vi "3_AdvancedDemo_MHT3.vi"() -> ()   [LabVIEW 2010]
uses:
  Types/MH_UIThread_Cmds.ctl
  _lib/PQ/MultiHarp/MH_InitInfo.ctl
  Types/MH_UIThread_Data.ctl
  Types/MH_InputChannel.ctl
  _lib/PQ/MultiHarp/MH_RefSource.ctl
  _lib/PQ/MultiHarp/mhlib_x86_x64_UIThread.llb/MH_DllPath_global.vi
  <vilib>/Utility/error.llb/DialogType.ctl
  Types/MH_DataProcThread_QCmds.ctl
  Types/MH_DataProcThread_QData.ctl
  Types/MH_VisThread_QCmds.ctl
  Types/MH_VisThread_QData.ctl
  Types/MH_VisThread_Data.ctl
  _lib/PQ/MultiHarp/MH_LibVersion_global.vi
  _lib/PQ/MultiHarp/MH_MeasMode.ctl
  Types/MH_SetInpChanData.ctl
  Types/MH_SetInpChanCmds.ctl
panel:
  in  "Settings":bool=TRUE
  in  "Run continuously":bool caption="Conti."
  in  "Start":bool
  in  "Scale":bool
  out "CountRates":i32[](graph)
  in  "AllChannels":T1={"Enable"=TRUE, "Offset"=0, "Level"=-100, "Edge"=0, "DeadTime"=1000, "UseDeadTime"=FALSE, "SetEnableAllChan"=TRUE, "SetEdgeAllChan"=TRUE, "SetLevelAllChan"=TRUE, "SetOffsetAllChan"=TRUE, "SetUseDTAllChan"=TRUE, "SetDeadTAllChan"=TRUE} {"DeadTime" min=800 max=160000 step=1; "Edge" items=["falling", "rising"]; "Offset" min=-100000 max=100000 step=5; "Level" min=-1200 max=1200 step=1}
  in  "HistoAcqTime":dbl=1.0 caption="Hist.Int.Time  s" min=0.1 max=360000.0 step=0.1
  in  "AcqTime":i32=360000000 caption="T3Acqu.       ms" min=1 max=360000 step=1
  in  "Binning":i32(ring) caption="Resol.            ps" items=["5", "10", "20", "40", "80", "160", "320", "640", "1280", "2560", "5120", "10240", "20480", "40960", "81920", "163840", "327680", "655360", "1310720", "2621440", "5242880", "10485760", "20971520", "41943040"]
  in  "HistoOffset":i32 caption="Offset            ns" min=0 max=100000000 step=1
  out "DeltaT":dbl=2.0479769602591973 caption="T.Tr.Resol.   ms" format="%.2f"
  in  "BitShift":i32=15 min=0 max=32 step=1
  in  "OvlLevel":u32=4294967295 caption="Ovl.Level" min=1024 max=65536 step=1024
  in  "StopOvl.":bool=TRUE
  out "TTraceGraph":T2(graph)={49.38852226226715, "Resolution"=0.00655367864414373, "Histogram"=[]}
  out "HistoGraph":cluster{dbl, "Resol":dbl, "Histos":u32[][]}(graph)={0.0, "Resol"=0.08, "Histos"=[]}
  in  "SyncDeadTime":i32=1000 caption="Dead T.   ps" min=800 max=160000 step=1
  in  "UseDeadTime":bool caption="Use DT."
  in  "SyncEdge":i32(ring) caption="Edge" items=["falling", "rising"]
  in  "SyncDivider":i32(ring) caption="Divider" items=["1", "2", "4", "8", "16"]
  in  "SyncOffset":i32 caption="Offset      ps" min=-100000 max=100000 step=5
  in  "SyncLevel":i32=-100 caption="Level      mV" min=-1200 max=1200 step=1
  in  "Channels":T3[](array[typedef])=[{"Name"="Inp.Chan 1", "Enable"=TRUE, "Edge"=0, "Level"=-100, "Offset"=0, "UseDeadTime"=FALSE, "DeadTime"=1000}, {"Name"="Inp.Chan 2", "Enable"=TRUE, "Edge"=0, "Level"=-100, "Offset"=0, "UseDeadTime"=FALSE, "DeadTime"=1000}, {"Name"="Inp.Chan 3", "Enable"=TRUE, "Edge"=0, "Level"=-100, "Offset"=0, "UseDeadTime"=FALSE, "DeadTime"=1000}, {"Name"="Inp.Chan 4", "Enable"=TRUE, "Edge"=0, "Level"=-100, "Offset"=0, "UseDeadTime"=FALSE, "DeadTime"=1000}, {"Name"="Inp.Chan 5", "Enable"=TRUE, "Edge"=0, "Level"=-100, "Offset"=0, "UseDeadTime"=FALSE, "DeadTime"=1000}, {"Name"="Inp.Chan 6", "Enable"=TRUE, "Edge"=0, "Level"=-100, "Offset"=0, "UseDeadTime"=FALSE, "DeadTime"=1000}, {"Name"="Inp.Chan 7", "Enable"=TRUE, "Edge"=0, "Level"=-100, "Offset"=0, "UseDeadTime"=FALSE, "DeadTime"=1000}, {"Name"="Inp.Chan 8", "Enable"=TRUE, "Edge"=0, "Level"=-100, "Offset"=0, "UseDeadTime"=FALSE, "DeadTime"=1000}, {"Name"="Inp.Chan 9", "Enable"=TRUE, "Edge"=0, "Level"=-100, "Offset"=0, "UseDeadTime"=FALSE, "DeadTime"=1000}, {"Name"="Inp.Chan 10", "Enable"=TRUE, "Edge"=0, "Level"=-100, "Offset"=0, "UseDeadTime"=FALSE, "DeadTime"=1000}, {"Name"="Inp.Chan 11", "Enable"=TRUE, "Edge"=0, "Level"=-100, "Offset"=0, "UseDeadTime"=FALSE, "DeadTime"=1000}, {"Name"="Inp.Chan 12", "Enable"=TRUE, "Edge"=0, "Level"=-100, "Offset"=0, "UseDeadTime"=FALSE, "DeadTime"=1000}, {"Name"="Inp.Chan 13", "Enable"=TRUE, "Edge"=0, "Level"=-100, "Offset"=0, "UseDeadTime"=FALSE, "DeadTime"=1000}, {"Name"="Inp.Chan 14", "Enable"=TRUE, "Edge"=0, "Level"=-100, "Offset"=0, "UseDeadTime"=FALSE, "DeadTime"=1000}, {"Name"="Inp.Chan 15", "Enable"=TRUE, "Edge"=0, "Level"=-100, "Offset"=0, "UseDeadTime"=FALSE, "DeadTime"=1000}, {"Name"="Inp.Chan 16", "Enable"=TRUE, "Edge"=0, "Level"=-100, "Offset"=0, "UseDeadTime"=FALSE, "DeadTime"=1000}, {"Name"="Inp.Chan 17", "Enable"=TRUE, "Edge"=0, "Level"=-100, "Offset"=0, "UseDeadTime"=FALSE, "DeadTime"=1000}, {"Name"="Inp.Chan 18", "Enable"=TRUE, "Edge"=0, "Level"=-100, "Offset"=0, "UseDeadTime"=FALSE, "DeadTime"=1000}, {"Name"="Inp.Chan 19", "Enable"=TRUE, "Edge"=0, "Level"=-100, "Offset"=0, "UseDeadTime"=FALSE, "DeadTime"=1000}, {"Name"="Inp.Chan 20", "Enable"=TRUE, "Edge"=0, "Level"=-100, "Offset"=0, "UseDeadTime"=FALSE, "DeadTime"=1000}, {"Name"="Inp.Chan 21", "Enable"=TRUE, "Edge"=0, "Level"=-100, "Offset"=0, "UseDeadTime"=FALSE, "DeadTime"=1000}, {"Name"="Inp.Chan 22", "Enable"=TRUE, "Edge"=0, "Level"=-100, "Offset"=0, "UseDeadTime"=FALSE, "DeadTime"=1000}, {"Name"="Inp.Chan 23", "Enable"=TRUE, "Edge"=0, "Level"=-100, "Offset"=0, "UseDeadTime"=FALSE, "DeadTime"=1000}, {"Name"="Inp.Chan 24", "Enable"=TRUE, "Edge"=0, "Level"=-100, "Offset"=0, "UseDeadTime"=FALSE, "DeadTime"=1000}, {"Name"="Inp.Chan 25", "Enable"=TRUE, "Edge"=0, "Level"=-100, "Offset"=0, "UseDeadTime"=FALSE, "DeadTime"=1000}, {"Name"="Inp.Chan 26", "Enable"=TRUE, "Edge"=0, "Level"=-100, "Offset"=0, "UseDeadTime"=FALSE, "DeadTime"=1000}, {"Name"="Inp.Chan 27", "Enable"=TRUE, "Edge"=0, "Level"=-100, "Offset"=0, "UseDeadTime"=FALSE, "DeadTime"=1000}, {"Name"="Inp.Chan 28", "Enable"=TRUE, "Edge"=0, "Level"=-100, "Offset"=0, "UseDeadTime"=FALSE, "DeadTime"=1000}, {"Name"="Inp.Chan 29", "Enable"=TRUE, "Edge"=0, "Level"=-100, "Offset"=0, "UseDeadTime"=FALSE, "DeadTime"=1000}, {"Name"="Inp.Chan 30", "Enable"=TRUE, "Edge"=0, "Level"=-100, "Offset"=0, "UseDeadTime"=FALSE, "DeadTime"=1000}, {"Name"="Inp.Chan 31", "Enable"=TRUE, "Edge"=0, "Level"=-100, "Offset"=0, "UseDeadTime"=FALSE, "DeadTime"=1000}, {"Name"="Inp.Chan 32", "Enable"=TRUE, "Edge"=0, "Level"=-100, "Offset"=0, "UseDeadTime"=FALSE, "DeadTime"=1000}, {"Name"="Inp.Chan 33", "Enable"=TRUE, "Edge"=0, "Level"=-100, "Offset"=0, "UseDeadTime"=FALSE, "DeadTime"=1000}, {"Name"="Inp.Chan 34", "Enable"=TRUE, "Edge"=0, "Level"=-100, "Offset"=0, "UseDeadTime"=FALSE, "DeadTime"=1000}, {"Name"="Inp.Chan 35", "Enable"=TRUE, "Edge"=0, "Level"=-100, "Offset"=0, "UseDeadTime"=FALSE, "DeadTime"=1000}, {"Name"="Inp.Chan 36", "Enable"=TRUE, "Edge"=0, "Level"=-100, "Offset"=0, "UseDeadTime"=FALSE, "DeadTime"=1000}, {"Name"="Inp.Chan 37", "Enable"=TRUE, "Edge"=0, "Level"=-100, "Offset"=0, "UseDeadTime"=FALSE, "DeadTime"=1000}, {"Name"="Inp.Chan 38", "Enable"=TRUE, "Edge"=0, "Level"=-100, "Offset"=0, "UseDeadTime"=FALSE, "DeadTime"=1000}, {"Name"="Inp.Chan 39", "Enable"=TRUE, "Edge"=0, "Level"=-100, "Offset"=0, "UseDeadTime"=FALSE, "DeadTime"=1000}, {"Name"="Inp.Chan 40", "Enable"=TRUE, "Edge"=0, "Level"=-100, "Offset"=0, "UseDeadTime"=FALSE, "DeadTime"=1000}, {"Name"="Inp.Chan 41", "Enable"=TRUE, "Edge"=0, "Level"=-100, "Offset"=0, "UseDeadTime"=FALSE, "DeadTime"=1000}, {"Name"="Inp.Chan 42", "Enable"=TRUE, "Edge"=0, "Level"=-100, "Offset"=0, "UseDeadTime"=FALSE, "DeadTime"=1000}, {"Name"="Inp.Chan 43", "Enable"=TRUE, "Edge"=0, "Level"=-100, "Offset"=0, "UseDeadTime"=FALSE, "DeadTime"=1000}, {"Name"="Inp.Chan 44", "Enable"=TRUE, "Edge"=0, "Level"=-100, "Offset"=0, "UseDeadTime"=FALSE, "DeadTime"=1000}, {"Name"="Inp.Chan 45", "Enable"=TRUE, "Edge"=0, "Level"=-100, "Offset"=0, "UseDeadTime"=FALSE, "DeadTime"=1000}, {"Name"="Inp.Chan 46", "Enable"=TRUE, "Edge"=0, "Level"=-100, "Offset"=0, "UseDeadTime"=FALSE, "DeadTime"=1000}, {"Name"="Inp.Chan 47", "Enable"=TRUE, "Edge"=0, "Level"=-100, "Offset"=0, "UseDeadTime"=FALSE, "DeadTime"=1000}, {"Name"="Inp.Chan 48", "Enable"=TRUE, "Edge"=0, "Level"=-100, "Offset"=0, "UseDeadTime"=FALSE, "DeadTime"=1000}, {"Name"="Inp.Chan 49", "Enable"=TRUE, "Edge"=0, "Level"=-100, "Offset"=0, "UseDeadTime"=FALSE, "DeadTime"=1000}, {"Name"="Inp.Chan 50", "Enable"=TRUE, "Edge"=0, "Level"=-100, "Offset"=0, "UseDeadTime"=FALSE, "DeadTime"=1000}, {"Name"="Inp.Chan 51", "Enable"=TRUE, "Edge"=0, "Level"=-100, "Offset"=0, "UseDeadTime"=FALSE, "DeadTime"=1000}, {"Name"="Inp.Chan 52", "Enable"=TRUE, "Edge"=0, "Level"=-100, "Offset"=0, "UseDeadTime"=FALSE, "DeadTime"=1000}, {"Name"="Inp.Chan 53", "Enable"=TRUE, "Edge"=0, "Level"=-100, "Offset"=0, "UseDeadTime"=FALSE, "DeadTime"=1000}, {"Name"="Inp.Chan 54", "Enable"=TRUE, "Edge"=0, "Level"=-100, "Offset"=0, "UseDeadTime"=FALSE, "DeadTime"=1000}, {"Name"="Inp.Chan 55", "Enable"=TRUE, "Edge"=0, "Level"=-100, "Offset"=0, "UseDeadTime"=FALSE, "DeadTime"=1000}, {"Name"="Inp.Chan 56", "Enable"=TRUE, "Edge"=0, "Level"=-100, "Offset"=0, "UseDeadTime"=FALSE, "DeadTime"=1000}, {"Name"="Inp.Chan 57", "Enable"=TRUE, "Edge"=0, "Level"=-100, "Offset"=0, "UseDeadTime"=FALSE, "DeadTime"=1000}, {"Name"="Inp.Chan 58", "Enable"=TRUE, "Edge"=0, "Level"=-100, "Offset"=0, "UseDeadTime"=FALSE, "DeadTime"=1000}, {"Name"="Inp.Chan 59", "Enable"=TRUE, "Edge"=0, "Level"=-100, "Offset"=0, "UseDeadTime"=FALSE, "DeadTime"=1000}, {"Name"="Inp.Chan 60", "Enable"=TRUE, "Edge"=0, "Level"=-100, "Offset"=0, "UseDeadTime"=FALSE, "DeadTime"=1000}, {"Name"="Inp.Chan 61", "Enable"=TRUE, "Edge"=0, "Level"=-100, "Offset"=0, "UseDeadTime"=FALSE, "DeadTime"=1000}, {"Name"="Inp.Chan 62", "Enable"=TRUE, "Edge"=0, "Level"=-100, "Offset"=0, "UseDeadTime"=FALSE, "DeadTime"=1000}, {"Name"="Inp.Chan 63", "Enable"=TRUE, "Edge"=0, "Level"=-100, "Offset"=0, "UseDeadTime"=FALSE, "DeadTime"=1000}, {"Name"="Inp.Chan 64", "Enable"=TRUE, "Edge"=0, "Level"=-100, "Offset"=0, "UseDeadTime"=FALSE, "DeadTime"=1000}] {"DeadTime" min=800 max=160000 step=1; "Edge" items=["falling", "rising"]; "Offset" min=-100000 max=100000 step=5; "Level" min=-1200 max=1200 step=1}
  out "SyncRate":string="Sync Rate: 16000190 cps\n"
  out "OverRun":bool caption="Overrun:"
  out "Status":string="Elements in Q: 0"
  # "All Channels"
  # "Acquisition"
  # "Sync"
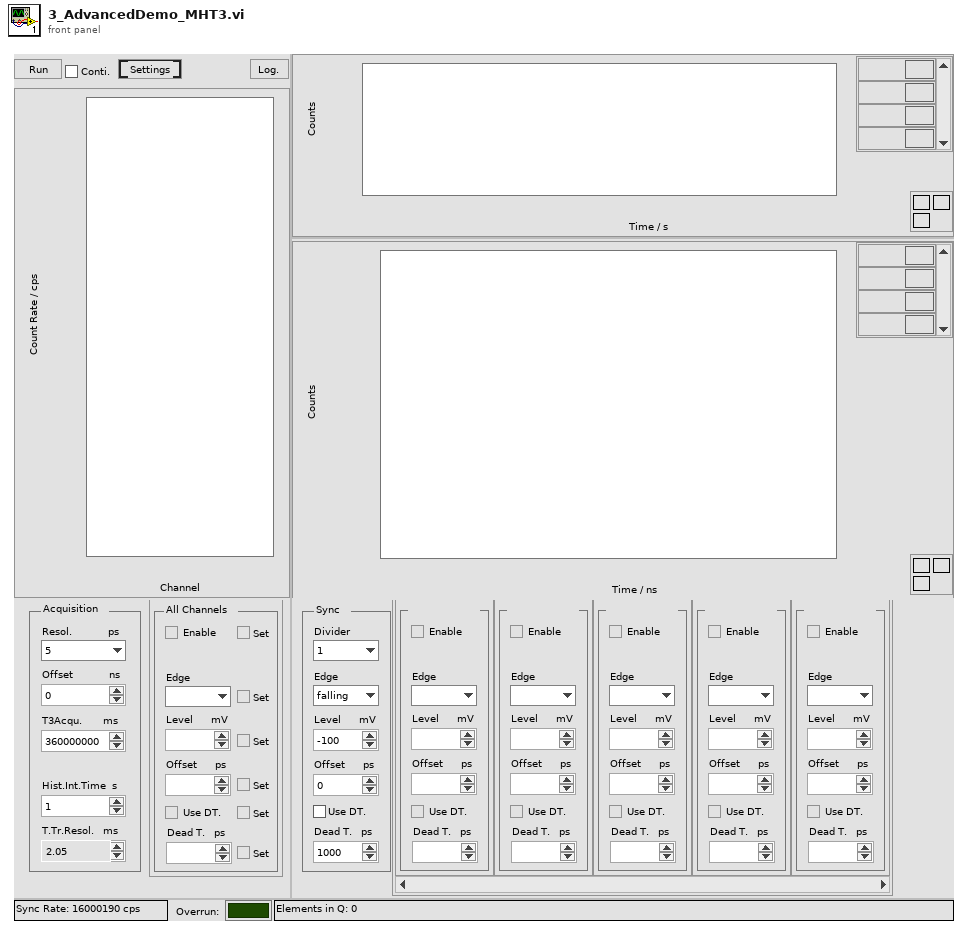
[diagram p1: front panel]
types:
  T1 = cluster{"Enable":bool, "Offset":i32, "Level":i32, "Edge":i32, "DeadTime":i32, "UseDeadTime":bool, "SetEnableAllChan":bool, "SetEdgeAllChan":bool, "SetLevelAllChan":bool, "SetOffsetAllChan":bool, "SetUseDTAllChan":bool, "SetDeadTAllChan":bool}
  T2 = cluster{dbl, "Resolution":dbl, "Histogram":u32[][]}
  T3 = typedef "MH_InputChannel.ctl" = cluster{"Name":string, "Enable":bool, "Edge":i32, "Level":i32, "Offset":i32, "UseDeadTime":bool, "DeadTime":i32}
  T4 = typedef "MH_DataProcThread_QCmds.ctl" = enum16{"Exit", "Proc", "Init", "SetShift", "SetNumChannels", "SetHistAcqTime"}
  T5 = typedef "MH_VisThread_Data.ctl" = cluster{"Resol":dbl, "DeltaT":dbl, "NumChannels":i32}
  T6 = typedef "MH_VisThread_QData.ctl" = cluster{"Histos":u32[][], "Cmd":T7, "TimeTrace":u32[][], "Bin":i32, "Total bin":u64, "Status":string, "Resol":dbl, "DeltaT":dbl, "nChannels":i32}
  T7 = typedef "MH_VisThread_QCmds.ctl" = enum16{"_none_", "Resol", "nChannels", "DeltaT", "Histo", "TTrace", "Status"}
  T8 = typedef "MH_DataProcThread_QData.ctl" = cluster{"Cmd":T4, "nActual":i32, "Buffer":u32[], "TickCount":u32, "Param":i32}
  T9 = typedef "MH_UIThread_Data.ctl" = cluster{"Init Info":T10, "DevIdx":i32, "SyncDivider":i32, "SyncOffset":i32, "SyncLevel":i32, "Channels":T3[], "CurrentChannels":i32[], "AcqTime":i32, "Binning":i32, "HistoOffset":i32, "HistoLen":i32, "StopOvl.":bool, "OvlLevel":u32, "SyncEdge":i32, "StartMeas":bool, "HistoLength":i32, "Resolution":dbl, "Run cont.":bool, "Status":string, "SyncRate":i32, "BitShift":i32, "HistoAcqTime":dbl, "SyncRateStart":i32, "UseDeadTime":bool, "SyncDeadTime":i32, "SetInpChan":T11[]}
  T10 = typedef "MH_InitInfo.ctl" = cluster{"Library Version":string, "Serial No.":string, "Model":string, "Partnum":string, "Version":string, "features":i32, "nchannels":i32, "Base Resolution":dbl, "Bin Steps":i32}
  T11 = typedef "MH_SetInpChanData.ctl" = cluster{"Channel":i32, "Cmds":T12[], "Changed":cluster{"Name":bool, "Enable":bool, "Edge":bool, "Level":bool, "Offset":bool, "UseDeadTime":bool, "DeadTime":bool}}
  T12 = typedef "MH_SetInpChanCmds.ctl" = enum16{"SetInpChanEnable", "SetInpChanOffset", "SetInpChanDeadTime", "SetInpChanTrg"}
  T13 = typedef "MH_UIThread_Cmds.ctl" = enum16{"Idle", "Init", "SetInpChan", "SetSyncDivider", "SetSyncTrg", "SetSyncOffset", "SetSyncDeadTime", "SetBinning", "SetHistoOffset", "SetHistoLen", "SetStopOvl", "SetBitShift", "SetHistoAcqTime", "GetRates", "GetAllRates", "StartMeas", "StopMeas", "AbortMeas", "GetResolution", "GetHistos", "GetAllHistos", "ReadFiFo", "WriteStatus", "Resize", "EnableControls", "DisableControls", "Error", "Exit"}
  T14 = enum8{"Enabled", "Disabled", "Disabled and Grayed Out"}
  T15 = cluster{"[0]":bool, "[1]":bool, "[2]":bool, "[3]":bool, "[4]":bool, "[5]":bool}
  T16 = typedef "MH_MeasMode.ctl" = i32
  T17 = typedef "MH_RefSource.ctl" = enum16{"INTERNAL", "EXTERNAL_10MHZ", "WR_MASTER_GENERIC", "WR_SLAVE_GENERIC", "WR_GRANDM_GENERIC", "EXTN_GPS_PPS", "EXTN_GPS_PPS_UART", "WR_MASTER_MHARP", "WR_SLAVE_MHARP", "WR_GRANDM_MHARP"}
  T18 = typedef "DialogType.ctl" = u16
  T19 = cluster{"T0":dbl, "dt":dbl, "TimeTrace_out":u32[][]}
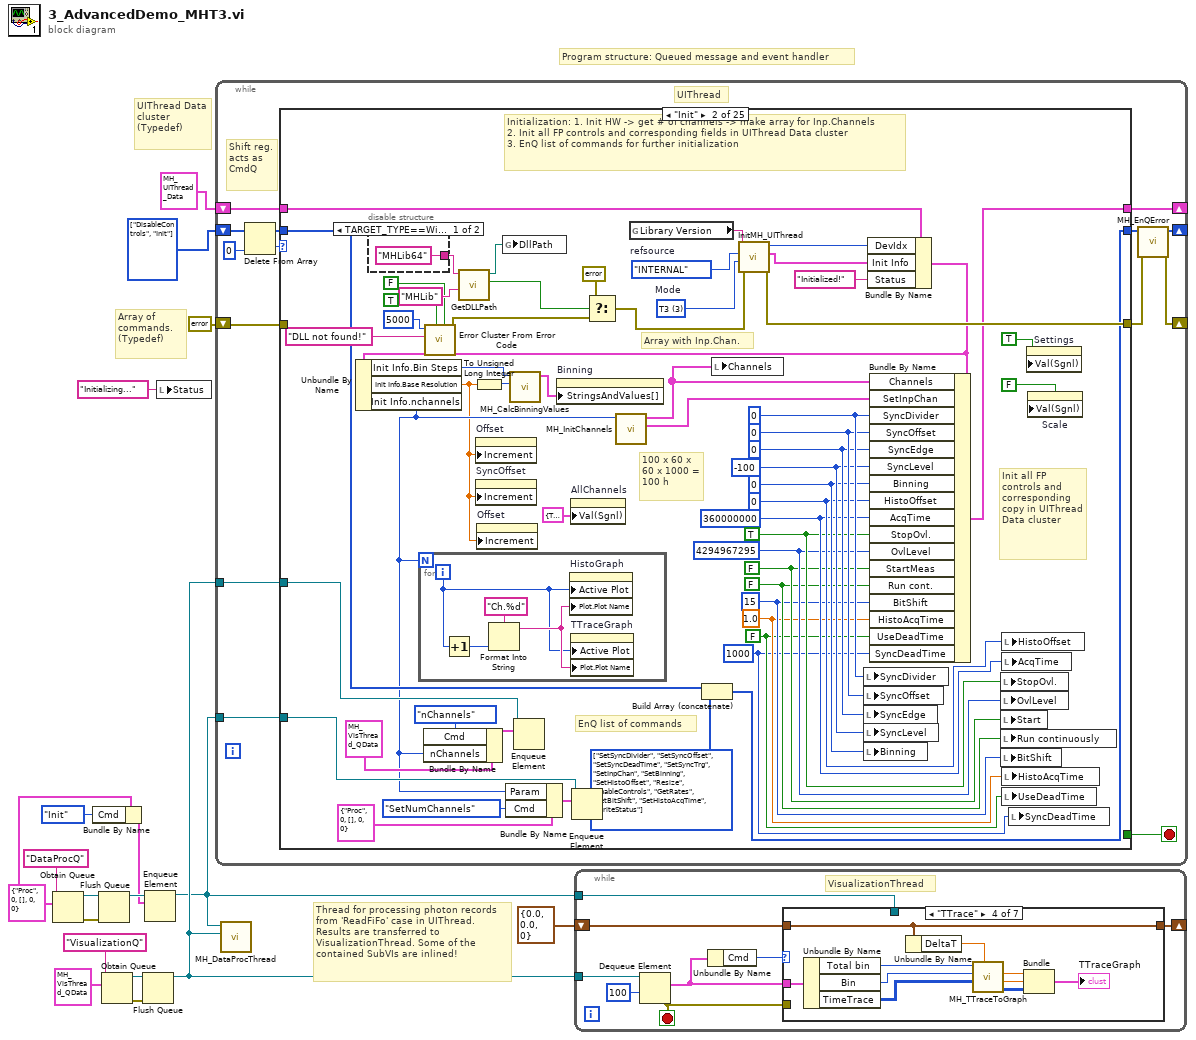
[diagram p0: block diagram]
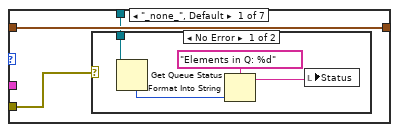
[diagram p2: hidden frame]
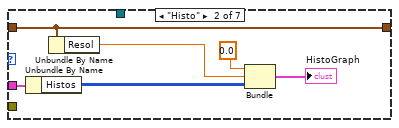
[diagram p4: hidden frame]
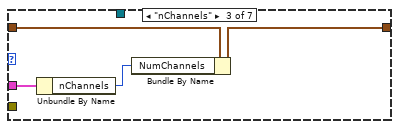
[diagram p5: hidden frame]
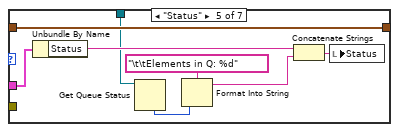
[diagram p6: hidden frame]
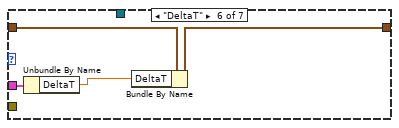
[diagram p7: hidden frame]
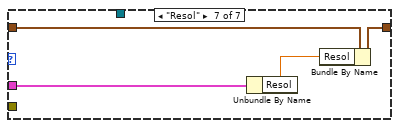
[diagram p8: hidden frame]
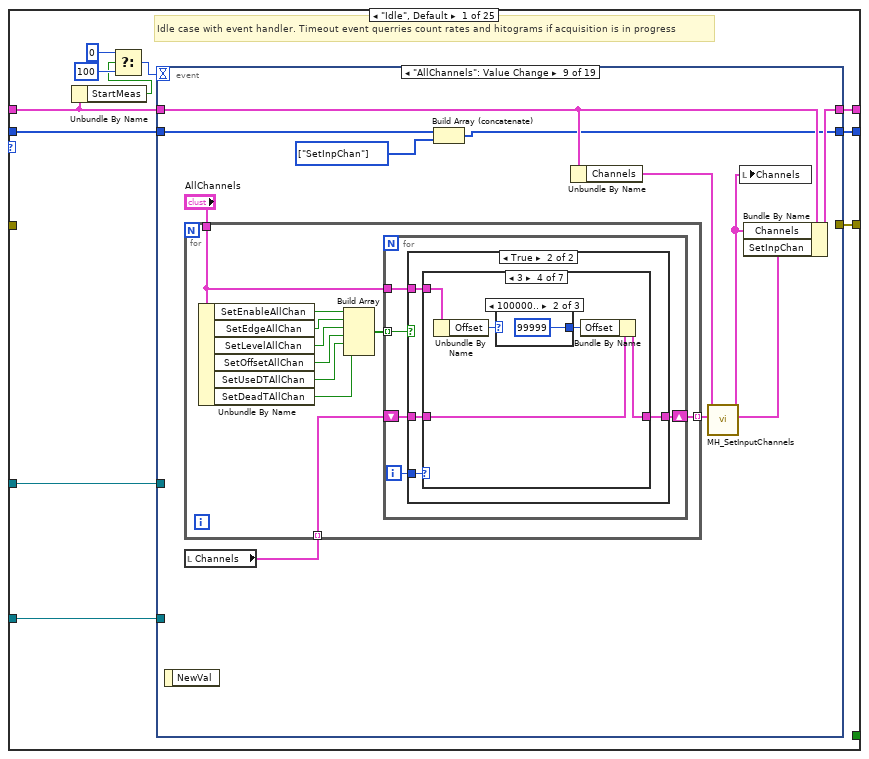
[diagram p9: hidden frame]
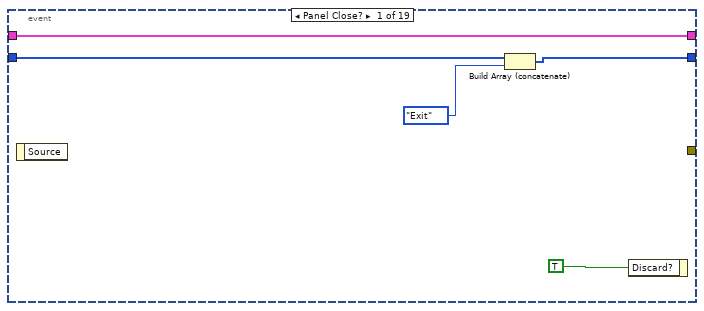
[diagram p10: hidden frame]
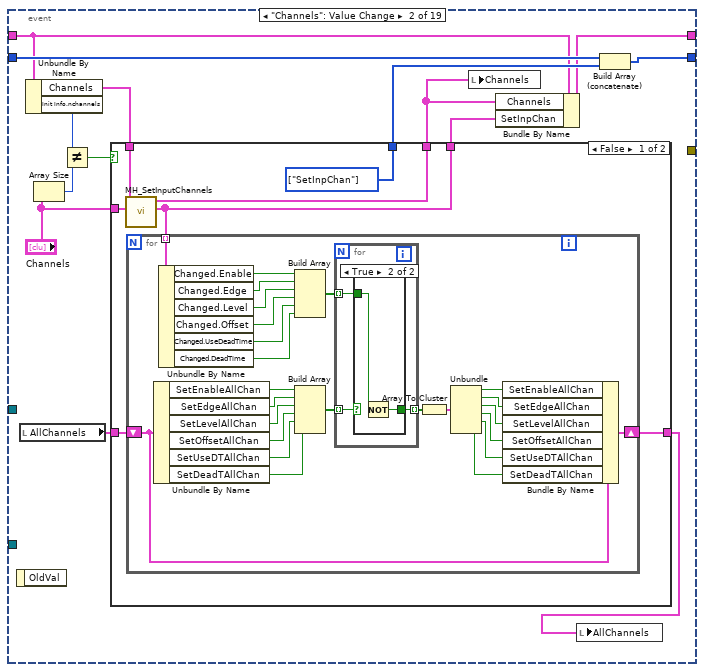
[diagram p11: hidden frame]
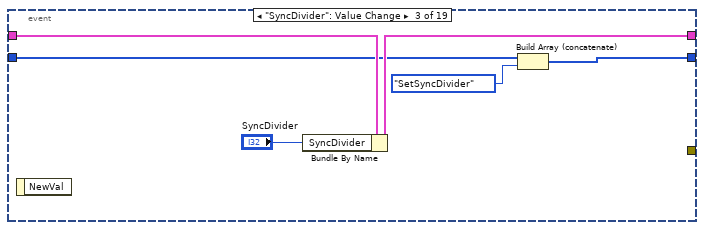
[diagram p14: hidden frame]
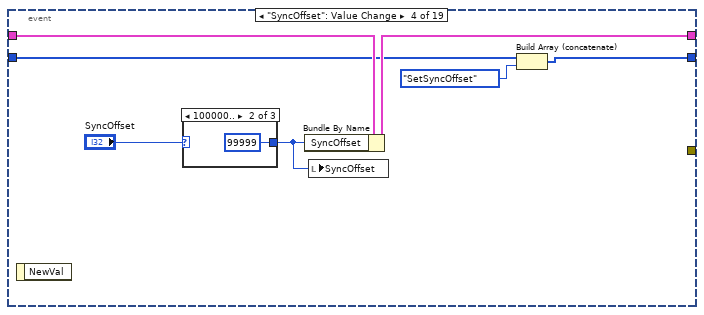
[diagram p15: hidden frame]
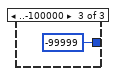
[diagram p17: hidden frame]
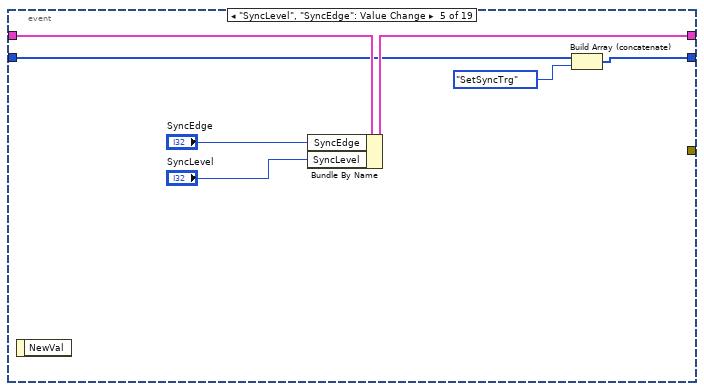
[diagram p18: hidden frame]
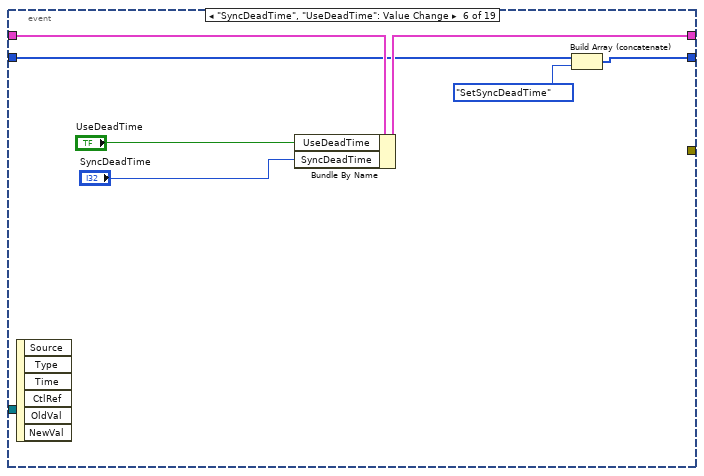
[diagram p19: hidden frame]
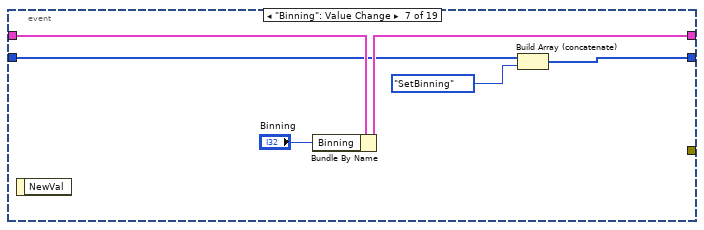
[diagram p20: hidden frame]
diagram:
  w4 = T8 {"Cmd"=enum."Proc", "nActual"=0, "Buffer"=[], "TickCount"=0, "Param"=0} ("MH_DataProcThread_QData")
  w17 = T13[] [enum."DisableControls", enum."Init"] items=["Idle", "Init", "SetInpChan", "SetSyncDivider", "SetSyncTrg", "SetSyncOffset", "SetSyncDeadTime", "SetBinning", "SetHistoOffset", "SetHistoLen", "SetStopOvl", "SetBitShift", "SetHistoAcqTime", "GetRates", "GetAllRates", "StartMeas", "StopMeas", "AbortMeas", "GetResolution", "GetHistos", "GetAllHistos", "ReadFiFo", "WriteStatus", "Resize", "EnableControls", "DisableControls", "Error", "Exit"]
  # "Thread for processing photon records from 'ReadFiFo' case in UIThread. Results are transferred to VisualizationThread. Some of the contained SubVIs are inlined!"
  # "Array of commands.\n(Typedef)"
  # "Program structure: Queued message and event handler"
  # "UIThread Data cluster\n(Typedef)"
  n1 = Obtain Queue(name (unnamed)="DataProcQ", element data type=w4) -> (queue out=w14:refnum<queue>, error out=w13:errorcluster)  [unwired: 3 in, 1 out]
  n2 = Bundle By Name(cluster=w4, "Cmd"=MH_DataProcThread_QCmds."Init") -> (w2:T8)
  n3 = Flush Queue(queue=w14, error in (no error)=w13) -> (queue out=w5:refnum<queue>)  [unwired: 2 out]
  n4 = Obtain Queue(name (unnamed)="VisualizationQ", element data type=T6 {"Histos"=[], "Cmd"=enum."_none_", "TimeTrace"=[], "Bin"=0, "Total bin"=0, "Status"="", "Resol"=0.0, "DeltaT"=0.0, "nChannels"=0} ("MH_GUIThread_QData")) -> (queue out=w12:refnum<queue>, error out=w11:errorcluster)  [unwired: 3 in, 1 out]
  n5 = Flush Queue(queue=w12, error in (no error)=w11) -> (queue out=w7:refnum<queue>)  [unwired: 2 out]
  n6 = Enqueue Element(queue=w5, element=w2) -> (queue out=w1:refnum<queue>)  [unwired: 2 in, 2 out]
  n7 = local write "Status"("Initializing..." ("Status")) -> ()
  n8 = while {
    shift-right: [w21] -> _
    shift-left: w17 -> [w28]
    shift-right: [w31] -> _
    shift-left: T9 {"Init Info"={"Library Version"="", "Serial No."="", "Model"="", "Partnum"="", "Version"="", "features"=0, "nchannels"=0, "Base Resolution"=0.0, "Bin Steps"=0}, "DevIdx"=0, "SyncDivider"=1, "SyncOffset"=0, "SyncLevel"=50, "Channels"=[], "CurrentChannels"=[], "AcqTime"=1, "Binning"=1, "HistoOffset"=1, "HistoLen"=1024, "StopOvl."=FALSE, "OvlLevel"=1024, "SyncEdge"=10, "StartMeas"=FALSE, "HistoLength"=0, "Resolution"=0.0, "Run cont."=FALSE, "Status"="", "SyncRate"=0, "BitShift"=0, "HistoAcqTime"=0.0, "SyncRateStart"=0, "UseDeadTime"=FALSE, "SyncDeadTime"=800, "SetInpChan"=[]} -> [w30]
    shift-right: [w23] -> _
    shift-left: errorcluster {"status"=FALSE, "code"=0, "source"=""} ("error IO") -> [w29]
    tunnel: w1 -> [w20]
    tunnel: w7 -> [w19]
    stop <- w32 stop-if-true
    # "Shift reg.\nacts as\nCmdQ"
    # "UIThread"
    n9 = Delete From Array(array=w28, index=0) -> (deleted portion=w26:T13, array with subset deleted=w25:T13[])  [unwired: 1 in]
    n10 = case shown="\"Init\"" w26 {
      tunnel: [w43 w359 w377 w439 w448 w460 w466 w473 w481 w488 w508 w520 w523 w595 w618 w623 w636 w653 w654 w680 w693 w700 w712 w718 w724] -> w22
      tunnel: [_ _ _ _ _ _ _ _ _ _ _ _ _ _ _ _ _ _ _ _ _ _ _ _ TRUE] -> w32
      tunnel: [w42 w340 w378 w441 w449 w461 w470 w477 w482 w489 w493 w510 w532 w587 w610 w626 w638 w649 w664 w679 w681 w699 w711 w719 w727] -> w31
      tunnel: w30 -> [w39 w345 w378 w441 w449 w461 w470 w477 w482 w489 w493 w510 w522 w588 w611 w627 w639 w650 w664 w679 w681 w699 w711 w719 w727]
      tunnel: [w40 w362 w372 w437 w447 w459 w469 w476 w480 w487 _ _ w528 w594 w621 w629 w641 w651 w659 _ _ _ _ _ w725] -> w24
      tunnel: w29 -> [_ _ _ _ _ _ _ _ _ _ _ _ _ _ _ _ _ _ _ _ _ _ _ w720 _]
      tunnel: w25 -> [w41 w361 w377 w439 w448 w460 w466 w472 w481 w488 w508 w520 w524 w595 w619 w624 w636 w653 w655 w680 w693 w700 w712 _ w724]
      tunnel: w20 -> [w34 w338 _ _ _ _ _ _ _ _ w494 w511 _ _ w615 _ _ _ w656 _ _ _ _ _ w723]
      tunnel: w19 -> [w33 w331 _ _ _ _ _ _ _ _ w495 _ _ _ _ _ _ w646 _ _ _ _ _ _ w722]
      frame "Idle", Default {
        # "Idle case with event handler. Timeout event querries count rates and hitograms if acquisition is in progress"
        n11 = Unbundle By Name(w39) -> ("StartMeas"=w37:bool)
        n12 = Select(t=0, s=w37, f=100) -> (s? t:f=w36:i32)
        n13 = event shown="[8] \"AllChannels\": Value Change" {
          selector: _ -> [_ _ _ _ _ _ _ _ _ _ _ _ _ _ _ _ _ _ _]
          dyn-events: _ -> [_ _ _ _ _ _ _ _ _ _ _ _ _ _ _ _ _ _ _]
          timeout: w36 -> [_ _ _ _ _ _ _ _ _ _ _ _ _ _ _ _ _ _ _]
          tunnel: [w44 w61 w103 w111 w120 w128 w134 w140 w145 w205 w210 w217 w232 w250 w262 w280 w286 w294 w304] -> w43
          tunnel: [w47 w53 w107 w114 w124 w131 w137 w143 w150 w207 w213 w220 w231 w254 w261 w278 w285 w293 w307] -> w42
          tunnel: w39 -> [w47 w54 w108 w115 w125 w132 w138 w144 w151 w208 w214 w221 w231 w255 w259 w279 w285 w293 w307]
          tunnel: w41 -> [w46 w62 w105 w113 w122 w130 w136 w142 w146 w205 w211 w219 w233 w251 w263 w280 w286 w294 w305]
          tunnel: [_ _ _ _ _ _ _ _ _ _ _ _ w227 _ _ _ _ _ _] -> w40
          tunnel: w34 -> [_ _ _ _ _ _ _ _ _ _ _ _ _ _ _ _ _ _ _]
          tunnel: w33 -> [_ _ _ _ _ _ _ _ _ _ _ _ _ _ _ _ _ _ _]
          event Panel Close? {
            n14 = event-data() -> ()  [unwired: 1 in, 1 out]
            n15 = Build Array (concatenate)(w46, MH_UIThread_Cmds."Exit") -> (w44:T13[])
            n16 = event-data("Discard?"=TRUE) -> ()  [unwired: 1 in, 1 out]
          }
          event "Channels": Value Change {
            n17 = event-data() -> ()  [unwired: 1 in, 1 out]
            n18 = local read "AllChannels"() -> (w49:T1)
            n19 = Unbundle By Name(w54) -> ("Channels"=w56:T3[], "Init Info.nchannels"=w58:i32)
            n20 = Array Size(array="Channels") -> (size(s)=w59:i32)
            n21 = Not Equal?(x=w58, y=w59) -> (x != y?=w57:bool)
            n22 = case shown="False" w57 {
              tunnel: "Channels" -> [w68 _]
              tunnel: [w67 w102] -> w51
              tunnel: w56 -> [w69 w102]
              tunnel: [w65 _] -> w52
              tunnel: [w66 _] -> w55
              tunnel: w49 -> [w64 w101]
              tunnel: [w63 w101] -> w50
              frame False {
                w66 = T13[] [enum."SetInpChan"] items=["Idle", "Init", "SetInpChan", "SetSyncDivider", "SetSyncTrg", "SetSyncOffset", "SetSyncDeadTime", "SetBinning", "SetHistoOffset", "SetHistoLen", "SetStopOvl", "SetBitShift", "SetHistoAcqTime", "GetRates", "GetAllRates", "StartMeas", "StopMeas", "AbortMeas", "GetResolution", "GetHistos", "GetAllHistos", "ReadFiFo", "WriteStatus", "Resize", "EnableControls", "DisableControls", "Error", "Exit"] ("array")
                n23 = call "MH_SetInputChannels.vi"("Channels new"=w68, "Channels old"=w69) -> ("SetInpChan"=w65:T11[], "Channels"=w67:T3[])  [unwired: 8 in]
                n24 = for {
                  tunnel: w65 -> [w94] mode=indexing
                  shift-right: [w76] -> w63
                  shift-left: w64 -> [w78]
                  n25 = Unbundle By Name(w78) -> ("SetEnableAllChan"=w87:bool, "SetEdgeAllChan"=w86:bool, "SetLevelAllChan"=w85:bool, "SetOffsetAllChan"=w84:bool, "SetUseDTAllChan"=w83:bool, "SetDeadTAllChan"=w82:bool)
                  n26 = Unbundle By Name(w94) -> ("Changed.Enable"=w93:bool, "Changed.Edge"=w92:bool, "Changed.Level"=w91:bool, "Changed.Offset"=w90:bool, "Changed.UseDeadTime"=w89:bool, "Changed.DeadTime"=w88:bool)
                  n27 = Build Array(w93, w92, w91, w90, w89, w88) -> (w80:bool[])
                  n28 = Build Array(w87, w86, w85, w84, w83, w82) -> (w81:bool[])
                  n29 = for {
                    tunnel: w81 -> [w97] mode=indexing
                    tunnel: w80 -> [w95] mode=indexing
                    tunnel: [w96] -> w79 mode=indexing
                    n30 = case shown="True" w97 {
                      selector: w97 -> [w98 _]
                      tunnel: [w98 w99] -> w96
                      tunnel: w95 -> [_ w100]
                      frame False {
                      }
                      frame True {
                        n31 = Not(x=w100) -> (.not. x?=w99:bool)
                      }
                    }
                  }
                  n32 = Array To Cluster(array=w79) -> (cluster=w77:T15)
                  n33 = Unbundle(w77) -> ("[0]"=w75:bool, "[1]"=w74:bool, "[2]"=w73:bool, "[3]"=w72:bool, "[4]"=w71:bool, "[5]"=w70:bool)
                  n34 = Bundle By Name(cluster=w78, "SetEnableAllChan"=w75, "SetEdgeAllChan"=w74, "SetLevelAllChan"=w73, "SetOffsetAllChan"=w72, "SetUseDTAllChan"=w71, "SetDeadTAllChan"=w70) -> (w76:T1)
                }
              }
              frame True {
              }
            }
            n35 = local write "Channels"(w51) -> ()
            n36 = Bundle By Name(cluster=w54, "Channels"=w51, "SetInpChan"=w52) -> (w53:T9)
            n37 = local write "AllChannels"(w50) -> ()
            n38 = Build Array (concatenate)(w62, w55) -> (w61:T13[])
          }
          event "SyncDivider": Value Change {
            n39 = event-data() -> ()  [unwired: 1 in, 1 out]
            n40 = Bundle By Name(cluster=w108, "SyncDivider"="SyncDivider") -> (w107:T9)
            n41 = Build Array (concatenate)(w105, MH_UIThread_Cmds."SetSyncDivider") -> (w103:T13[])
          }
          event "SyncOffset": Value Change {
            n42 = event-data() -> ()  [unwired: 1 in, 1 out]
            n43 = case shown="100000.." "SyncOffset" {
              selector: "SyncOffset" -> [w116 _ _]
              tunnel: [w116 99999 ("SyncOffset") -99999 ("SyncOffset")] -> w109
              frame Default {
              }
              frame 100000.. {
              }
              frame ..-100000 {
              }
            }
            n44 = Bundle By Name(cluster=w115, "SyncOffset"=w109) -> (w114:T9)
            n45 = local write "SyncOffset"(w109) -> ()
            n46 = Build Array (concatenate)(w113, MH_UIThread_Cmds."SetSyncOffset") -> (w111:T13[])
          }
          event "SyncLevel", "SyncEdge": Value Change {
            n47 = event-data() -> ()  [unwired: 1 in, 1 out]
            n48 = Bundle By Name(cluster=w125, "SyncEdge"="SyncEdge", "SyncLevel"="SyncLevel") -> (w124:T9)
            n49 = Build Array (concatenate)(w122, MH_UIThread_Cmds."SetSyncTrg") -> (w120:T13[])
          }
          event "SyncDeadTime", "UseDeadTime": Value Change {
            n50 = event-data() -> ()  [unwired: 1 in, 6 out]
            n51 = Bundle By Name(cluster=w132, "UseDeadTime"="UseDeadTime", "SyncDeadTime"="SyncDeadTime") -> (w131:T9)
            n52 = Build Array (concatenate)(w130, MH_UIThread_Cmds."SetSyncDeadTime") -> (w128:T13[])
          }
          event "Binning": Value Change {
            n53 = event-data() -> ()  [unwired: 1 in, 1 out]
            n54 = Bundle By Name(cluster=w138, "Binning"="Binning") -> (w137:T9)
            n55 = Build Array (concatenate)(w136, MH_UIThread_Cmds."SetBinning") -> (w134:T13[])
          }
          event "HistoOffset": Value Change {
            n56 = event-data() -> ()  [unwired: 1 in, 1 out]
            n57 = Bundle By Name(cluster=w144, "HistoOffset"="HistoOffset") -> (w143:T9)
            n58 = Build Array (concatenate)(w142, MH_UIThread_Cmds."SetHistoOffset") -> (w140:T13[])
          }
          event "AllChannels": Value Change {
            w147 = T13[] [enum."SetInpChan"] items=["Idle", "Init", "SetInpChan", "SetSyncDivider", "SetSyncTrg", "SetSyncOffset", "SetSyncDeadTime", "SetBinning", "SetHistoOffset", "SetHistoLen", "SetStopOvl", "SetBitShift", "SetHistoAcqTime", "GetRates", "GetAllRates", "StartMeas", "StopMeas", "AbortMeas", "GetResolution", "GetHistos", "GetAllHistos", "ReadFiFo", "WriteStatus", "Resize", "EnableControls", "DisableControls", "Error", "Exit"] ("array")
            n59 = event-data() -> ()  [unwired: 1 in, 1 out]
            n60 = local read "Channels"() -> (w154:T3[])
            n61 = for {
              tunnel: w154 -> [w158] mode=indexing
              tunnel: "AllChannels" -> [w157]
              tunnel: [w156] -> w153 mode=indexing
              n62 = Unbundle By Name(w157) -> ("SetEnableAllChan"=w159:bool, "SetEdgeAllChan"=w160:bool, "SetLevelAllChan"=w161:bool, "SetOffsetAllChan"=w162:bool, "SetUseDTAllChan"=w163:bool, "SetDeadTAllChan"=w164:bool)
              n63 = Build Array(w159, w160, w161, w162, w163, w164) -> (w165:bool[])
              n64 = for {
                tunnel: w165 -> [w170] mode=indexing
                shift-right: [w167] -> w156
                shift-left: w158 -> [w168]
                tunnel: w157 -> [w166]
                i -> [w169]
                n65 = case shown="True" w170 {
                  tunnel: w169 -> [_ w175]
                  tunnel: w166 -> [_ w174]
                  tunnel: w168 -> [w171 w173]
                  tunnel: [w171 w172] -> w167
                  frame False {
                  }
                  frame True {
                    n66 = case shown="3" w175 {
                      tunnel: w174 -> [w179 w183 w187 w192 w199 w203 _]
                      tunnel: w173 -> [w178 w182 w186 w191 w198 w202 w204]
                      tunnel: [w176 w180 w184 w190 w196 w200 w204] -> w172
                      frame 0 {
                        n67 = Unbundle By Name(w179) -> ("Enable"=w177:bool)
                        n68 = Bundle By Name(cluster=w178, "Enable"=w177) -> (w176:T3)
                      }
                      frame 1 {
                        n69 = Unbundle By Name(w183) -> ("Edge"=w181:i32)
                        n70 = Bundle By Name(cluster=w182, "Edge"=w181) -> (w180:T3)
                      }
                      frame 2 {
                        n71 = Unbundle By Name(w187) -> ("Level"=w185:i32)
                        n72 = Bundle By Name(cluster=w186, "Level"=w185) -> (w184:T3)
                      }
                      frame 3 {
                        n73 = Unbundle By Name(w192) -> ("Offset"=w189:i32)
                        n74 = case shown="100000.." w189 {
                          selector: w189 -> [w193 _ _]
                          tunnel: [w193 99999 ("SyncOffset") -99999 ("SyncOffset")] -> w188
                          frame Default {
                          }
                          frame 100000.. {
                          }
                          frame ..-100000 {
                          }
                        }
                        n75 = Bundle By Name(cluster=w191, "Offset"=w188) -> (w190:T3)
                      }
                      frame 4 {
                        n76 = Unbundle By Name(w199) -> ("UseDeadTime"=w197:bool)
                        n77 = Bundle By Name(cluster=w198, "UseDeadTime"=w197) -> (w196:T3)
                      }
                      frame 5 {
                        n78 = Unbundle By Name(w203) -> ("DeadTime"=w201:i32)
                        n79 = Bundle By Name(cluster=w202, "DeadTime"=w201) -> (w200:T3)
                      }
                      frame Default {
                      }
                    }
                  }
                }
              }
            }
            n80 = Build Array (concatenate)(w146, w147) -> (w145:T13[])
            n81 = Unbundle By Name(w151) -> ("Channels"=w152:T3[])
            n82 = call "MH_SetInputChannels.vi"("Channels new"=w153, "Channels old"=w152) -> ("SetInpChan"=w148:T11[], "Channels"=w149:T3[])  [unwired: 8 in]
            n83 = local write "Channels"(w149) -> ()
            n84 = Bundle By Name(cluster=w151, "Channels"=w149, "SetInpChan"=w148) -> (w150:T9)
          }
          event "AcqTime": Value Change {
            n85 = event-data() -> ()  [unwired: 1 in, 1 out]
            n86 = Bundle By Name(cluster=w208, "AcqTime"="AcqTime") -> (w207:T9)
          }
          event "HistoAcqTime": Value Change {
            n87 = event-data() -> ()  [unwired: 1 in, 1 out]
            n88 = Bundle By Name(cluster=w214, "HistoAcqTime"="HistoAcqTime") -> (w213:T9)
            n89 = Build Array (concatenate)(w211, MH_UIThread_Cmds."SetHistoAcqTime") -> (w210:T13[])
          }
          event "OvlLevel", "StopOvl.": Value Change {
            n90 = event-data() -> ()  [unwired: 1 in, 1 out]
            n91 = Bundle By Name(cluster=w221, "StopOvl."="StopOvl.", "OvlLevel"="OvlLevel") -> (w220:T9)
            n92 = Build Array (concatenate)(w219, MH_UIThread_Cmds."SetStopOvl") -> (w217:T13[])
          }
          event Timeout {
            n93 = event-data() -> ()  [unwired: 1 in, 1 out]
            n94 = Unbundle By Name(w231) -> ("DevIdx"=w229:i32, "StartMeas"=w230:bool, "BitShift"=w226:i32, "SyncRate"=w225:i32)
            n95 = case shown="True" w230 {
              tunnel: w229 -> [_ w249]
              tunnel: [_ w247] -> w228
              tunnel: [_ w244] -> w227
              frame False {
              }
              frame True {
                w245 = T13[] [enum."ReadFiFo"] items=["Idle", "Init", "SetInpChan", "SetSyncDivider", "SetSyncTrg", "SetSyncOffset", "SetSyncDeadTime", "SetBinning", "SetHistoOffset", "SetHistoLen", "SetStopOvl", "SetBitShift", "SetHistoAcqTime", "GetRates", "GetAllRates", "StartMeas", "StopMeas", "AbortMeas", "GetResolution", "GetHistos", "GetAllHistos", "ReadFiFo", "WriteStatus", "Resize", "EnableControls", "DisableControls", "Error", "Exit"]
                w246 = T13[] [enum."StopMeas"] items=["Idle", "Init", "SetInpChan", "SetSyncDivider", "SetSyncTrg", "SetSyncOffset", "SetSyncDeadTime", "SetBinning", "SetHistoOffset", "SetHistoLen", "SetStopOvl", "SetBitShift", "SetHistoAcqTime", "GetRates", "GetAllRates", "StartMeas", "StopMeas", "AbortMeas", "GetResolution", "GetHistos", "GetAllHistos", "ReadFiFo", "WriteStatus", "Resize", "EnableControls", "DisableControls", "Error", "Exit"]
                n96 = call "MH_CTCStatus.vi"("devidx"=w249) -> ("error out"=w244:errorcluster, "ctcstatus"=w248:i32)  [unwired: 8 in, 1 out]
                n97 = Not Equal To 0?(x=w248) -> (x != 0?=w243:bool)
                n98 = Select(t=w246, s=w243, f=w245) -> (s? t:f=w247:T13[])
              }
            }
            n99 = call "CalcRate.vi"("Refresh(ms)"=u32 100) -> ("updated?"=w223:bool)  [unwired: 8 in, 2 out]
            n100 = case shown="True" w223 {
              tunnel: w226 -> [_ w236]
              tunnel: w225 -> [_ w235]
              tunnel: [_ MH_UIThread_Cmds."GetAllRates"] -> w224
              frame False {
              }
              frame True {
                n101 = To Double Precision Float(number=w235) -> (double precision float=w240:dbl)
                n102 = To Double Precision Float(number=w236) -> (double precision float=w241:dbl)
                n103 = Power Of 2(x=w241) -> (2^x=w239:dbl)
                n104 = Multiply(x=w239, y=1000.0) -> (x*y=w238:dbl)
                n105 = Divide(x=w238, y=w240) -> (x/y=w242:dbl)
                n106 = local write "DeltaT"(w242) -> ()
              }
            }
            n107 = Build Array (concatenate)(w233, w228, w224) -> (w232:T13[])
          }
          event "BitShift": Value Change {
            n108 = event-data() -> ()  [unwired: 1 in, 1 out]
            n109 = Bundle By Name(cluster=w255, "BitShift"="BitShift") -> (w254:T9)
            n110 = Build Array (concatenate)(w251, MH_UIThread_Cmds."SetBitShift") -> (w250:T13[])
          }
          event "Start": Value Change {
            n111 = event-data() -> ()  [unwired: 1 in, 1 out]
            n112 = Unbundle By Name(w259) -> ("SyncRate"=w258:i32)
            n113 = Greater Or Equal?(x=w258, y=10) -> (x >= y?=w256:bool)
            n114 = case shown="True" w256 {
              selector: w256 -> [w265 _]
              tunnel: w263 -> [w267 w276]
              tunnel: [w267 w274] -> w262
              tunnel: [w266 w273] -> w261
              tunnel: "Start" -> [_ w272]
              tunnel: w259 -> [w266 w268]
              frame False {
                n115 = local write "Start"(w265) -> ()
                n116 = One Button Dialog(message="SyncRate too low!!!" ("Status")) -> ()  [unwired: 1 in, 1 out]
              }
              frame True {
                w271 = T13[] [enum."SetBitShift", enum."SetHistoAcqTime", enum."StartMeas"] items=["Idle", "Init", "SetInpChan", "SetSyncDivider", "SetSyncTrg", "SetSyncOffset", "SetSyncDeadTime", "SetBinning", "SetHistoOffset", "SetHistoLen", "SetStopOvl", "SetBitShift", "SetHistoAcqTime", "GetRates", "GetAllRates", "StartMeas", "StopMeas", "AbortMeas", "GetResolution", "GetHistos", "GetAllHistos", "ReadFiFo", "WriteStatus", "Resize", "EnableControls", "DisableControls", "Error", "Exit"]
                n117 = Bundle By Name(cluster=w268, "StartMeas"=w272) -> (w273:T9)
                n118 = Build Array(MH_UIThread_Cmds."AbortMeas") -> (w269:T13[])
                n119 = Select(t=w271, s=w272, f=w269) -> (s? t:f=w275:T13[])
                n120 = Build Array (concatenate)(w276, w275) -> (w274:T13[])
              }
            }
          }
          event "Run continuously": Value Change {
            n121 = event-data() -> ()  [unwired: 1 in, 1 out]
            n122 = Bundle By Name(cluster=w279, "Run cont."="Run continuously") -> (w278:T9)
          }
          event "Scale": Value Change {
            n123 = event-data() -> ()  [unwired: 1 in, 1 out]
            n124 = Select(t=u8 0 ("Y Scale.Mapping Mode"), s="Scale", f=u8 1 ("Y Scale.Mapping Mode")) -> (s? t:f=w281:u8)
            n125 = property on="HistoGraph" class="WFGraph (strict)"("YScale.Mapping Mode"=w281) -> ()  [unwired: 2 in, 2 out]
          }
          event "Settings": Value Change {
            n126 = event-data() -> ()  [unwired: 1 in, 1 out]
            n127 = property on="Splitter" class="Splitter"() -> ("Position"=w292:i32)  [unwired: 2 in, 2 out]
            n128 = Select(t=300 ("PosT"), s="Settings", f=0 ("PosF")) -> (s? t:f=w289:i32)
            n129 = Subtract(x=w292, y=w289) -> (x-y=w288:i32)
            n130 = while {
              shift-right: [w303] -> _
              shift-left: w288 -> [w296]
              i -> [w302]
              stop <- w299 stop-if-true
              n131 = property on="Splitter 4" class="Splitter"("Position"=w296) -> (error out=w295:errorcluster)  [unwired: 2 in, 1 out]
              n132 = Greater Or Equal?(x=w302, y=10) -> (x >= y?=w300:bool)
              n133 = Decrement(x=w296) -> (x-1=w303:i32)
              n134 = Unbundle(w295) -> ("status"=w298:bool)  [unwired: 2 out]
              n135 = Not(x=w298) -> (.not. x?=w297:bool)
              n136 = Or(x=w297, y=w300) -> (x .or. y?=w299:bool)
            }
          }
          event Panel Resize {
            n137 = event-data() -> ()  [unwired: 1 in, 1 out]
            n138 = Build Array (concatenate)(w305, MH_UIThread_Cmds."Resize") -> (w304:T13[])
          }
        }
      }
      frame "Init" {
        w318 = 1000 ("SyncDeadTime")
        w319 = FALSE ("UseDeadTime")
        w321 = T16 3 items=["HIST"=0, "T2"=2, "T3"=3]  # Mode
        w323 = MH_RefSource."INTERNAL"  # refsource
        w329 = 1.0 ("HistoAcqTime")
        w330 = 15 ("Value (Signaling)")
        w347 = FALSE ("Run cont.")
        w349 = FALSE ("StartMeas")
        w350 = u32 4294967295 ("OvlLevel")
        w351 = TRUE ("StopOvl.")
        w352 = 360000000 ("AcqTime")
        w353 = 0 ("HistoOffset")
        w354 = 0 ("Binning")
        w355 = -100 ("SyncLevel")
        w356 = 0 ("SyncZeroX")
        w357 = 0 ("SyncOffset")
        w358 = 0 ("SyncDivider")
        w360 = T13[] [enum."SetSyncDivider", enum."SetSyncOffset", enum."SetSyncDeadTime", enum."SetSyncTrg", enum."SetInpChan", enum."SetBinning", enum."SetHistoOffset", enum."Resize", enum."EnableControls", enum."GetRates", enum."SetBitShift", enum."SetHistoAcqTime", enum."WriteStatus"] items=["Idle", "Init", "SetInpChan", "SetSyncDivider", "SetSyncTrg", "SetSyncOffset", "SetSyncDeadTime", "SetBinning", "SetHistoOffset", "SetHistoLen", "SetStopOvl", "SetBitShift", "SetHistoAcqTime", "GetRates", "GetAllRates", "StartMeas", "StopMeas", "AbortMeas", "GetResolution", "GetHistos", "GetAllHistos", "ReadFiFo", "WriteStatus", "Resize", "EnableControls", "DisableControls", "Error", "Exit"]
        # "100 x 60 x 60 x 1000 = 100 h"
        # "Init all FP controls and corresponding copy in UIThread Data cluster"
        # "EnQ list of commands"
        # "Array with Inp.Chan."
        # "Initialization: 1. Init HW -> get # of channels -> make array for Inp.Channels\n2. Init all FP controls and corresponding fields in UIThread Data cluster\n3. EnQ list of commands for further initialization"
        n139 = disable-structure shown="TARGET_TYPE==Windows, Default" {
          disable-tunnel: ["MHLib64" ("name or relative path") "MHLib" ("name or relative path")] -> w320
          frame condition #0 (active) {
          }
          frame condition #1 {
          }
        }
        n140 = call <vilib>:"Error Cluster From Error Code.vi"("is warning? (False)"=FALSE, "show call chain? (False)"=TRUE, "error message (\"\")"="DLL not found!" ("error message (\"\")"), "error code (0)"=5000) -> ("error out"=w324:errorcluster)  [unwired: 5 in]
        n141 = call "GetDLLPath.vi"("DllName_32bit"="MHLib" ("name or relative path"), "DllName_64bit"=w320) -> ("file exists?"=w326:bool, "DLLPath"=w327:path)  [unwired: 8 in]
        n142 = global write "MH_DllPath_global.vi" "DllPath"(w327) -> ()
        n143 = property on="AllChannels" class="Clust (strict)"("Val(Sgnl)"=T1 {"Enable"=TRUE, "Offset"=0, "Level"=-100, "Edge"=0, "DeadTime"=1000, "UseDeadTime"=FALSE, "SetEnableAllChan"=TRUE, "SetEdgeAllChan"=TRUE, "SetLevelAllChan"=TRUE, "SetOffsetAllChan"=TRUE, "SetUseDTAllChan"=TRUE, "SetDeadTAllChan"=TRUE} ("AllChannels")) -> ()  [unwired: 2 in, 2 out]
        n144 = Select(t=errorcluster {"status"=FALSE, "code"=0, "source"=""} ("error IO"), s=w326, f=w324) -> (s? t:f=w341:errorcluster)
        n145 = global read "MH_LibVersion_global.vi" "Library Version"() -> (w322:string)
        n146 = Build Array (concatenate)(w361, w360) -> (w359:T13[])
        n147 = call "InitMH_UIThread.vi"("error in (no error)"=w341, "Mode"=w321, "refsource"=w323, "Library Version"=w322) -> ("error out"=w362:errorcluster, "Init Info"=w364:T10, "DevIdx"=w363:i32)  [unwired: 5 in]
        n148 = local write "SyncDivider"(w358) -> ()
        n149 = local write "SyncOffset"(w357) -> ()
        n150 = local write "SyncEdge"(w356) -> ()
        n151 = local write "SyncLevel"(w355) -> ()
        n152 = local write "Binning"(w354) -> ()
        n153 = Bundle By Name(cluster=w345, "DevIdx"=w363, "Init Info"=w364, "Status"="Initialized!") -> (w344:T9)
        n154 = Unbundle By Name(w344) -> ("Init Info.Bin Steps"=w343:i32, "Init Info.Base Resolution"=w312:dbl, "Init Info.nchannels"=w317:i32)
        n155 = for {
          N: w317 -> [_]
          i -> [w367]
          n156 = Increment(x=w367) -> (x+1=w370:i32)
          n157 = Format Into String(format string="Ch.%d", w370) -> (resulting string=w368:string)  [unwired: 2 in, 1 out]
          n158 = property on="HistoGraph" class="WFGraph (strict)"("Active Plot"=w367, "Plot.Plot Name"=w368) -> ()  [unwired: 2 in, 2 out]
          n159 = property on="TTraceGraph" class="WFGraph (strict)"("Active Plot"=w367, "Plot.Plot Name"=w368) -> ()  [unwired: 2 in, 2 out]
        }
        n160 = Bundle By Name(cluster=T6 {"Histos"=[], "Cmd"=enum."_none_", "TimeTrace"=[], "Bin"=0, "Total bin"=0, "Status"="", "Resol"=0.0, "DeltaT"=0.0, "nChannels"=0} ("MH_GUIThread_QData"), "Cmd"=MH_VisThread_QCmds."nChannels", "nChannels"=w317) -> (w333:T6)
        n161 = To Unsigned Long Integer(number=w312) -> (unsigned 32bit integer=w313:u32)
        n162 = property on="Offset" class="DigNum (strict)"("Increment"=w312) -> ()  [unwired: 2 in, 2 out]
        n163 = property on="SyncOffset" class="DigNum (strict)"("Increment"=w312) -> ()  [unwired: 2 in, 2 out]
        n164 = property on="Offset" class="DigNum (strict)"("Increment"=w312) -> ()  [unwired: 2 in, 2 out]
        n165 = Bundle By Name(cluster=T8 {"Cmd"=enum."Proc", "nActual"=0, "Buffer"=[], "TickCount"=0, "Param"=0} ("MH_DataProcThread_QData"), "Param"=w317, "Cmd"=MH_DataProcThread_QCmds."SetNumChannels") -> (w337:T8)
        n166 = call "MH_CalcBinningValues.vi"("BaseResolution"=w313, "Bin Steps"=w343) -> ("BinningValues"=w348:cluster{"String":string, "Value":i32}[])  [unwired: 9 in]
        n167 = Enqueue Element(queue=w331, element=w333) -> ()  [unwired: 2 in, 3 out]
        n168 = property on="Binning" class="Ring (strict)"("StringsAndValues[]"=w348) -> ()  [unwired: 2 in, 2 out]
        n169 = Enqueue Element(queue=w338, element=w337) -> ()  [unwired: 2 in, 3 out]
        n170 = call "MH_InitChannels.vi"("nchannels"=w317) -> ("SetInpChan"=w315:T11[], "Channels"=w316:T3[])  [unwired: 9 in]
        n171 = local write "Channels"(w316) -> ()
        n172 = Bundle By Name(cluster=w344, "Channels"=w316, "SetInpChan"=w315, "SyncDivider"=w358, "SyncOffset"=w357, "SyncEdge"=w356, "SyncLevel"=w355, "Binning"=w354, "HistoOffset"=w353, "AcqTime"=w352, "StopOvl."=w351, "OvlLevel"=w350, "StartMeas"=w349, "Run cont."=w347, "BitShift"=w330, "HistoAcqTime"=w329, "UseDeadTime"=w319, "SyncDeadTime"=w318) -> (w340:T9)
        n173 = local write "StopOvl."(w351) -> ()
        n174 = local write "OvlLevel"(w350) -> ()
        n175 = local write "Start"(w349) -> ()
        n176 = local write "Run continuously"(w347) -> ()
        n177 = local write "BitShift"(w330) -> ()
        n178 = local write "HistoOffset"(w353) -> ()
        n179 = local write "AcqTime"(w352) -> ()
        n180 = local write "HistoAcqTime"(w329) -> ()
        n181 = local write "UseDeadTime"(w319) -> ()
        n182 = local write "SyncDeadTime"(w318) -> ()
        n183 = property on="Settings" class="Bool (strict)"("Val(Sgnl)"=TRUE ("Value (Signaling)")) -> ()  [unwired: 2 in, 2 out]
        n184 = property on="Scale" class="Bool (strict)"("Val(Sgnl)"=FALSE ("Value (Signaling)")) -> ()  [unwired: 2 in, 2 out]
      }
      frame "SetInpChan" {
        n185 = Unbundle By Name(w378) -> ("DevIdx"=w376:i32, "Init Info.features"=w375:i32, "SetInpChan"=w374:T11[], "Channels"=w373:T3[])
        n186 = for {
          tunnel: w373 -> [w383]
          tunnel: w374 -> [w387] mode=indexing
          shift-right: [w385] -> w372
          shift-left: errorcluster {"status"=FALSE, "code"=0, "source"=""} ("error out") -> [w384]
          tunnel: w376 -> [w381]
          tunnel: w375 -> [w379]
          n187 = Unbundle By Name(w387) -> ("Cmds"=w386:T12[], "Channel"=w380:i32)
          n188 = Index Array(array=w383, index=w380) -> (element=w382:T3)
          n189 = for {
            tunnel: w386 -> [w394] mode=indexing
            tunnel: w380 -> [w393]
            shift-right: [w392] -> w385
            shift-left: w384 -> [w391]
            tunnel: w382 -> [w390]
            tunnel: w381 -> [w389]
            tunnel: w379 -> [w388]
            n190 = case shown="\"SetInpChanDeadTime\"" w394 {
              tunnel: w393 -> [_ w400 w407 w412 w428]
              tunnel: [w395 w399 w406 w416 w433] -> w392
              tunnel: w391 -> [w395 w398 w405 w415 w432]
              tunnel: w390 -> [_ w397 w404 w414 w431]
              tunnel: w389 -> [_ w396 w403 w413 w430]
              tunnel: w388 -> [_ _ _ w409 _]
              frame Default {
              }
              frame "SetInpChanEnable" {
                n191 = Unbundle By Name(w397) -> ("Enable"=w401:bool)
                n192 = call "MH_SetInputChannelEnable.vi"("error in (no error)"=w398, "enable"=w401, "channel"=w400, "devidx"=w396) -> ("error out"=w399:errorcluster)  [unwired: 6 in, 1 out]
              }
              frame "SetInpChanOffset" {
                n193 = Unbundle By Name(w404) -> ("Offset"=w402:i32)
                n194 = call "MH_SetInputChannelOffset.vi"("error in (no error)"=w405, "Offset"=w402, "channel"=w407, "devidx"=w403) -> ("error out"=w406:errorcluster)  [unwired: 6 in, 1 out]
              }
              frame "SetInpChanDeadTime" {
                w410 = 32  # FEATURE_PROG_TD
                n195 = And(x=w409, y=w410) -> (x .and. y?=w411:i32)
                n196 = Not Equal To 0?(x=w411) -> (x != 0?=w408:bool)
                n197 = case shown="False" w408 {
                  tunnel: [w417 w426] -> w416
                  tunnel: w415 -> [w417 w425]
                  tunnel: w414 -> [_ w424]
                  tunnel: w413 -> [_ w423]
                  tunnel: w412 -> [_ w421]
                  frame False {
                  }
                  frame True {
                    n198 = Unbundle By Name(w424) -> ("UseDeadTime"=w420:bool, "DeadTime"=w422:i32)
                    n199 = Boolean To (0,1)(Boolean=w420) -> (0, 1=w419:i16)
                    n200 = To Long Integer(number=w419) -> (32bit integer=w418:i32)
                    n201 = call "MH_SetInputDeadTime.vi"("channel"=w421, "error in (no error)"=w425, "deadtime"=w422, "on"=w418, "devidx"=w423) -> ("error out"=w426:errorcluster)  [unwired: 5 in, 1 out]
                  }
                }
              }
              frame "SetInpChanTrg" {
                n202 = Unbundle By Name(w431) -> ("Level"=w427:i32, "Edge"=w429:i32)
                n203 = call "MH_SetInputEdgeTrg.vi"("channel"=w428, "error in (no error)"=w432, "edge"=w429, "level"=w427, "devidx"=w430) -> ("error out"=w433:errorcluster)  [unwired: 5 in, 1 out]
              }
            }
          }
        }
      }
      frame "SetSyncDivider" {
        n204 = Unbundle By Name(w441) -> ("DevIdx"=w440:i32, "SyncDivider"=w436:i32)
        n205 = Power Of 2(x=w436) -> (2^x=w435:dbl)
        n206 = To Long Integer(number=w435) -> (32bit integer=w434:i32)
        n207 = call "MH_SetSyncDiv.vi"("SyncDivider"=w434, "devidx"=w440) -> ("error out"=w438:errorcluster)  [unwired: 8 in, 1 out]
        n208 = flat-sequence {
          tunnel: w438 -> [w442]
          tunnel: [w442] -> w437
          frame #0 {
            n209 = Wait (ms)(milliseconds to wait=u32 100) -> ()  [unwired: 1 out]
          }
        }
      }
      frame "SetSyncTrg" {
        n210 = Unbundle By Name(w449) -> ("DevIdx"=w446:i32, "SyncLevel"=w444:i32, "SyncEdge"=w445:i32)
        n211 = call "MH_SetSyncEdgeTrg.vi"("edge"=w445, "level"=w444, "devidx"=w446) -> ("error out"=w447:errorcluster)  [unwired: 7 in, 1 out]
      }
      frame "SetSyncDeadTime" {
        w452 = 32  # FEATURE_PROG_TD
        n212 = Unbundle By Name(w461) -> ("DevIdx"=w458:i32, "UseDeadTime"=w455:bool, "SyncDeadTime"=w457:i32, "Init Info.features"=w451:i32)
        n213 = And(x=w451, y=w452) -> (x .and. y?=w453:i32)
        n214 = Boolean To (0,1)(Boolean=w455) -> (0, 1=w456:i16)
        n215 = Not Equal To 0?(x=w453) -> (x != 0?=w450:bool)
        n216 = To Long Integer(number=w456) -> (32bit integer=w454:i32)
        n217 = case shown="True" w450 {
          tunnel: [_ w465] -> w459
          tunnel: w458 -> [_ w464]
          tunnel: w457 -> [_ w463]
          tunnel: w454 -> [_ w462]
          frame False {
          }
          frame True {
            n218 = call "MH_SetSyncDeadTime.vi"("deadtime"=w463, "on"=w462, "devidx"=w464) -> ("error out"=w465:errorcluster)  [unwired: 7 in, 1 out]
          }
        }
      }
      frame "SetSyncOffset" {
        n219 = Unbundle By Name(w470) -> ("DevIdx"=w468:i32, "SyncOffset"=w467:i32)
        n220 = call "MH_SetSyncChannelOffset.vi"("Offset"=w467, "devidx"=w468) -> ("error out"=w469:errorcluster)  [unwired: 8 in, 1 out]
      }
      frame "SetBinning" {
        # "When binning is changed the new resolution is querried"
        n221 = Unbundle By Name(w477) -> ("DevIdx"=w475:i32, "Binning"=w474:i32)
        n222 = call "MH_SetBinning.vi"("Binning"=w474, "devidx"=w475) -> ("error out"=w476:errorcluster)  [unwired: 8 in, 1 out]
        n223 = Build Array (concatenate)(MH_UIThread_Cmds."GetResolution", w472) -> (w473:T13[])
      }
      frame "SetHistoOffset" {
        n224 = Unbundle By Name(w482) -> ("DevIdx"=w479:i32, "HistoOffset"=w478:i32)
        n225 = call "MH_SetOffset.vi"("Offset"=w478, "devidx"=w479) -> ("error out"=w480:errorcluster)  [unwired: 8 in, 1 out]
      }
      frame "SetStopOvl" {
        n226 = Unbundle By Name(w489) -> ("DevIdx"=w486:i32, "StopOvl."=w485:bool, "OvlLevel"=w484:u32)
        n227 = To Unsigned Long Integer(number=w484) -> (unsigned 32bit integer=w483:u32)
        n228 = call "MH_SetStopOverflow.vi"("stopcount"=w483, "StopOnOverflow"=w485, "devidx"=w486) -> ("error out"=w487:errorcluster)  [unwired: 7 in, 1 out]
      }
      frame "SetBitShift" {
        n229 = Unbundle By Name(w493) -> ("BitShift"=w491:i32, "SyncRate"=w492:i32)
        n230 = Negate(x=w491) -> (-x=w501:i32)
        n231 = Bundle By Name(cluster=T8 {"Cmd"=enum."Proc", "nActual"=0, "Buffer"=[], "TickCount"=0, "Param"=0} ("MH_DataProcThread_QData"), "Param"=w501, "Cmd"=MH_DataProcThread_QCmds."SetShift") -> (w507:T8)
        n232 = To Double Precision Float(number=w491) -> (double precision float=w506:dbl)
        n233 = To Double Precision Float(number=w492) -> (double precision float=w505:dbl)
        n234 = Power Of 2(x=w506) -> (2^x=w504:dbl)
        n235 = Enqueue Element(queue=w494, element=w507) -> ()  [unwired: 2 in, 3 out]
        n236 = Multiply(x=w504, y=1000.0) -> (x*y=w503:dbl)
        n237 = Divide(x=w503, y=w505) -> (x/y=w490:dbl)
        "DeltaT" <- w490
        n238 = Bundle By Name(cluster=T6 {"Histos"=[], "Cmd"=enum."_none_", "TimeTrace"=[], "Bin"=0, "Total bin"=0, "Status"="", "Resol"=0.0, "DeltaT"=0.0, "nChannels"=0} ("MH_GUIThread_QData"), "DeltaT"=w490, "Cmd"=MH_VisThread_QCmds."DeltaT") -> (w502:T6)
        n239 = Enqueue Element(queue=w495, element=w502) -> ()  [unwired: 2 in, 3 out]
      }
      frame "SetHistoAcqTime" {
        n240 = Unbundle By Name(w510) -> ("SyncRate"=w516:i32, "HistoAcqTime"=w509:dbl)
        n241 = To Double Precision Float(number=w516) -> (double precision float=w519:dbl)
        n242 = Multiply(x=w519, y=w509) -> (x*y=w518:dbl)
        n243 = Round To Nearest(number=w518) -> (nearest integer value=w517:dbl)
        n244 = To Long Integer(number=w517) -> (32bit integer=w515:i32)
        n245 = Bundle By Name(cluster=T8 {"Cmd"=enum."Proc", "nActual"=0, "Buffer"=[], "TickCount"=0, "Param"=0} ("MH_DataProcThread_QData"), "Param"=w515, "Cmd"=MH_DataProcThread_QCmds."SetHistAcqTime") -> (w514:T8)
        n246 = Enqueue Element(queue=w511, element=w514) -> ()  [unwired: 2 in, 3 out]
      }
      frame "GetAllRates" {
        # "An alternative to GetRates"
        n247 = Unbundle By Name(w522) -> ("DevIdx"=w530:i32, "Init Info.nchannels"=w537:i32, "StartMeas"=w531:bool, "SyncRateStart"=w525:i32)
        n248 = call "MH_AllocateCntRateBuffer.vi"("NumChan"=w537) -> ("Buffer"=w536:i32[])  [unwired: 10 in]
        n249 = call "MH_GetAllCountRates.vi"("cntrates_buf"=w536, "devidx"=w530) -> ("error out"=w529:errorcluster, "cntrates"=→"CountRates":i32[], "syncrate"=w527:i32)  [unwired: 6 in, 1 out]
        n250 = case shown="True" w531 {
          tunnel: w530 -> [_ w552]
          tunnel: w529 -> [w541 w551]
          tunnel: [w541 w550] -> w528
          tunnel: w527 -> [w540 _]
          tunnel: [w540 w547] -> w526
          tunnel: w525 -> [_ w542]
          tunnel: w524 -> [w539 w546]
          tunnel: [w539 w545] -> w523
          tunnel: w522 -> [w538 w544]
          tunnel: [w538 w543] -> w521
          frame False {
          }
          frame True {
            n251 = call "MH_GetSyncPeriod.vi"("error in (no error)"=w551, "devidx"=w552) -> ("error out"=w550:errorcluster, "period"=w549:dbl)  [unwired: 7 in, 1 out]
            n252 = Reciprocal(x=w549) -> (1/x=w548:dbl)
            n253 = To Long Integer(number=w548) -> (32bit integer=w547:i32)
            n254 = case shown="-1" w542 {
              selector: w542 -> [w553 _ _]
              tunnel: w547 -> [w556 w577 _]
              tunnel: w546 -> [w554 w579 w583]
              tunnel: [w555 w579 w583] -> w545
              tunnel: w544 -> [w560 w578 w582]
              tunnel: [w560 w576 w581] -> w543
              frame Default {
                n255 = Subtract(x=w556, y=w553) -> (x-y=w559:i32)
                n256 = Absolute Value(x=w559) -> (abs(x)=w557:i32)
                n257 = Not Equal To 0?(x=w557) -> (x != 0?=w558:bool)
                n258 = case shown="True" w558 {
                  tunnel: w557 -> [_ w569]
                  tunnel: [w561 w564] -> w555
                  tunnel: w554 -> [w561 w563]
                  tunnel: w553 -> [_ w562]
                  frame False {
                  }
                  frame True {
                    n259 = To Double Precision Float(number=w569) -> (double precision float=w568:dbl)
                    n260 = To Double Precision Float(number=w562) -> (double precision float=w570:dbl)
                    n261 = Divide(x=w568, y=w570) -> (x/y=w567:dbl)
                    n262 = Greater Or Equal?(x=w567, y=0.01) -> (x >= y?=w565:bool)
                    n263 = case shown="False" w565 {
                      tunnel: [w571 w574] -> w564
                      tunnel: w563 -> [w571 w572]
                      frame False {
                      }
                      frame True {
                        w573 = T13[] [enum."StopMeas"] items=["Idle", "Init", "SetInpChan", "SetSyncDivider", "SetSyncTrg", "SetSyncOffset", "SetSyncDeadTime", "SetBinning", "SetHistoOffset", "SetHistoLen", "SetStopOvl", "SetBitShift", "SetHistoAcqTime", "GetRates", "GetAllRates", "StartMeas", "StopMeas", "AbortMeas", "GetResolution", "GetHistos", "GetAllHistos", "ReadFiFo", "WriteStatus", "Resize", "EnableControls", "DisableControls", "Error", "Exit"]
                        n264 = One Button Dialog(message="Warning: Sync Rate has changed!\nTime Trace resolution has been changed accordingly.\nMeasurement is aborted.\n") -> ()  [unwired: 1 in, 1 out]
                        n265 = Build Array (concatenate)(w572, w573) -> (w574:T13[])
                      }
                    }
                  }
                }
              }
              frame -1 {
                n266 = Bundle By Name(cluster=w578, "SyncRateStart"=w577) -> (w576:T9)
              }
              frame -2 {
                n267 = Bundle By Name(cluster=w582, "SyncRateStart"=-1) -> (w581:T9)
              }
            }
          }
        }
        n268 = Bundle By Name(cluster=w521, "SyncRate"=w526) -> (w532:T9)
        n269 = Format Into String(format string="Sync Rate: %d cps\n", w526) -> (resulting string=→"SyncRate":string)  [unwired: 2 in, 1 out]
      }
      frame "GetRates" {
        # "An alternative to GetAllRates"
        n270 = Unbundle By Name(w588) -> ("Init Info.nchannels"=w593:i32, "Channels"=w589:T3[], "DevIdx"=w590:i32)
        n271 = call "MH_GetSyncRate.vi"("devidx"=w590) -> ("error out"=w592:errorcluster, "syncrate"=w586:i32)  [unwired: 8 in, 1 out]
        n272 = Format Into String(format string="Sync Rate: %d cps\n", w586) -> (resulting string=w585:string)  [unwired: 2 in, 1 out]
        n273 = local write "SyncRate"(w585) -> ()
        n274 = for {
          N: w593 -> [_]
          tunnel: w590 -> [w601]
          tunnel: [w598] -> w584 mode=indexing
          shift-right: [w600] -> w594
          shift-left: w592 -> [w602]
          tunnel: w589 -> [w597] mode=indexing
          i -> [w599]
          n275 = Unbundle By Name(w597) -> ("Enable"=w596:bool)
          n276 = case shown="True" w596 {
            tunnel: w602 -> [w603 w608]
            tunnel: w601 -> [_ w607]
            tunnel: [w603 w606] -> w600
            tunnel: w599 -> [_ w605]
            tunnel: [_ w604] -> w598
            frame False {
            }
            frame True {
              n277 = call "MH_GetCountRate.vi"("error in (no error)"=w608, "Channel"=w605, "devidx"=w607) -> ("error out"=w606:errorcluster, "rate"=w604:i32)  [unwired: 6 in, 1 out]
            }
          }
        }
        n278 = local write "CountRates"(w584) -> ()
        n279 = Bundle By Name(cluster=w588, "SyncRate"=w586) -> (w587:T9)
      }
      frame "StartMeas" {
        n280 = Bundle By Name(cluster=T8 {"Cmd"=enum."Proc", "nActual"=0, "Buffer"=[], "TickCount"=0, "Param"=0} ("MH_DataProcThread_QData"), "Cmd"=MH_DataProcThread_QCmds."Init") -> (w613:T8)
        n281 = Unbundle By Name(w611) -> ("DevIdx"=w620:i32, "AcqTime"=w616:i32)
        n282 = Enqueue Element(queue=w615, element=w613) -> ()  [unwired: 2 in, 3 out]
        n283 = Bundle By Name(cluster=w611, "SyncRateStart"=-2) -> (w610:T9)
        n284 = call "MH_StartMeas.vi"("tacq"=w616, "devidx"=w620) -> ("error out"=w621:errorcluster)  [unwired: 8 in, 1 out]
        n285 = Build Array (concatenate)(w619, MH_UIThread_Cmds."ReadFiFo") -> (w618:T13[])
      }
      frame "StopMeas" {
        n286 = Unbundle By Name(w627) -> ("Run cont."=w622:bool, "DevIdx"=w628:i32)
        n287 = call "MH_StopMeas.vi"("devidx"=w628) -> ("error out"=w629:errorcluster)  [unwired: 9 in, 1 out]
        n288 = case shown="False" w622 {
          tunnel: w627 -> [w633 w635]
          tunnel: [w632 w635] -> w626
          tunnel: [w630 w634] -> w625
          frame False {
            w630 = T13[] [enum."ReadFiFo"] items=["Idle", "Init", "SetInpChan", "SetSyncDivider", "SetSyncTrg", "SetSyncOffset", "SetSyncDeadTime", "SetBinning", "SetHistoOffset", "SetHistoLen", "SetStopOvl", "SetBitShift", "SetHistoAcqTime", "GetRates", "GetAllRates", "StartMeas", "StopMeas", "AbortMeas", "GetResolution", "GetHistos", "GetAllHistos", "ReadFiFo", "WriteStatus", "Resize", "EnableControls", "DisableControls", "Error", "Exit"]
            w631 = FALSE ("StartMeas")
            n289 = Bundle By Name(cluster=w633, "StartMeas"=w631) -> (w632:T9)
            n290 = local write "Start"(w631) -> ()
          }
          frame True {
            w634 = T13[] [enum."ReadFiFo", enum."StartMeas"] items=["Idle", "Init", "SetInpChan", "SetSyncDivider", "SetSyncTrg", "SetSyncOffset", "SetSyncDeadTime", "SetBinning", "SetHistoOffset", "SetHistoLen", "SetStopOvl", "SetBitShift", "SetHistoAcqTime", "GetRates", "GetAllRates", "StartMeas", "StopMeas", "AbortMeas", "GetResolution", "GetHistos", "GetAllHistos", "ReadFiFo", "WriteStatus", "Resize", "EnableControls", "DisableControls", "Error", "Exit"]
          }
        }
        n291 = Build Array (concatenate)(w624, w625) -> (w623:T13[])
      }
      frame "AbortMeas" {
        w637 = FALSE ("StartMeas")
        n292 = Unbundle By Name(w639) -> ("DevIdx"=w640:i32)
        n293 = call "MH_StopMeas.vi"("devidx"=w640) -> ("error out"=w641:errorcluster)  [unwired: 9 in, 1 out]
        n294 = Bundle By Name(cluster=w639, "StartMeas"=w637) -> (w638:T9)
        n295 = local write "Start"(w637) -> ()
      }
      frame "GetResolution" {
        # "Resolution in ns"
        # "Gets resolution in ps"
        # "Resolution is saved in UIThread Data cluster in ns"
        n296 = Unbundle By Name(w650) -> ("DevIdx"=w652:i32)
        n297 = call "MH_GetResolution.vi"("devidx"=w652) -> ("error out"=w651:errorcluster, "resolution"=w648:dbl)  [unwired: 8 in, 1 out]
        n298 = Divide(x=w648, y=1000.0) -> (x/y=w644:dbl)
        n299 = Bundle By Name(cluster=w650, "Resolution"=w644) -> (w649:T9)
        n300 = Bundle By Name(cluster=T6 {"Histos"=[], "Cmd"=enum."_none_", "TimeTrace"=[], "Bin"=0, "Total bin"=0, "Status"="", "Resol"=0.0, "DeltaT"=0.0, "nChannels"=0} ("MH_GUIThread_QData"), "Resol"=w644, "Cmd"=MH_VisThread_QCmds."Resol") -> (w642:T6)
        n301 = Enqueue Element(queue=w646, element=w642) -> ()  [unwired: 2 in, 3 out]
      }
      frame "ReadFiFo" {
        w662 = 2  # FLAG_FIFOFULL
        # "Reads photon records from HW and transferes them to DataProcThread via Queue."
        n302 = Unbundle By Name(w664) -> ("DevIdx"=w658:i32)
        n303 = call "MH_GetFlags.vi"("devidx"=w658) -> ("error out"=w660:errorcluster, "flags"=w661:i32)  [unwired: 8 in, 1 out]
        n304 = And(x=w661, y=w662) -> (x .and. y?=w663:i32)
        n305 = Not Equal To 0?(x=w663) -> (x != 0?=w657:bool)
        "OverRun" <- w657
        n306 = case shown="False" w657 {
          tunnel: w660 -> [w674 w677]
          tunnel: [w673 w677] -> w659
          tunnel: w658 -> [w666 _]
          tunnel: w656 -> [w672 _]
          tunnel: w655 -> [w671 _]
          tunnel: [w671 w675] -> w654
          frame False {
            n307 = call "MH_ReadFiFo.vi"("error in (no error)"=w674, "devidx"=w666) -> ("error out"=w673:errorcluster, "nactual"=w665:i32, "buffer"=w669:u32[])  [unwired: 6 in, 1 out]
            n308 = Bundle By Name(cluster=T8 {"Cmd"=enum."Proc", "nActual"=0, "Buffer"=[], "TickCount"=0, "Param"=0} ("MH_DataProcThread_QData"), "Buffer"=w669, "nActual"=w665, "Cmd"=MH_DataProcThread_QCmds."Proc") -> (w667:T8)
            n309 = Enqueue Element(queue=w672, element=w667) -> ()  [unwired: 2 in, 3 out]
          }
          frame True {
            n310 = Build Array(MH_UIThread_Cmds."AbortMeas") -> (w675:T13[])
          }
        }
      }
      frame "WriteStatus" {
        n311 = Unbundle By Name(w679) -> ("Status"=→"Status":string)
      }
      frame "Resize" {
        n312 = property on="Pane 3" class="Pane"() -> ("Width"=w686:u32)  [unwired: 2 in, 2 out]
        n313 = Subtract(x=w686, y=i16 100 ("b")) -> (x-y=w692:u32)
        n314 = Unbundle By Name(w681) -> ("Init Info.nchannels"=w689:i32)
        n315 = Quotient & Remainder(x=w692, y=i16 99 ("m")) -> (floor(x/y)=w691:u32)  [unwired: 1 out]
        n316 = In Range and Coerce(upper limit=w689, x=w691, lower limit=4) -> (coerced(x)=w690:u32)  [unwired: 1 out]
        n317 = Equal?(x=w689, y=w690) -> (x = y?=w688:bool)
        n318 = Not(x=w688) -> (.not. x?=w687:bool)
        n319 = property on="Channels" class="Arr (strict)"("HorizScroll"=w687, "Number of Columns"=w690, "Index Values"=u32[] [0]) -> ()  [unwired: 2 in, 2 out]
      }
      frame "EnableControls" {
        n320 = property class="VI"() -> ("Panel"=w697:refnum<vi>)  [unwired: 2 in, 2 out]
        n321 = property class="Pnl"(reference=w697) -> ("Controls[]"=w696:refnum<vi>[])  [unwired: 1 in, 2 out]
        n322 = property class="Pnl"(reference=w697) -> ("Decos[]"=w698:refnum<vi>[])  [unwired: 1 in, 2 out]
        n323 = for {
          tunnel: w698 -> [w702] mode=indexing
          tunnel: TRUE -> [w701]
          n324 = property class="Decor"(reference=w702, "Visible"=w701) -> ()  [unwired: 1 in, 2 out]
        }
        n325 = for {
          tunnel: w696 -> [w705] mode=indexing
          tunnel: T14."Enabled" ("Disabled") -> [w704]
          tunnel: [w703] -> _
          n326 = property class="Ctl"(reference=w705, "DisabledEnum"=w704) -> (error out=w703:errorcluster)  [unwired: 1 in, 1 out]
        }
      }
      frame "DisableControls" {
        n327 = property class="VI"() -> ("Panel"=w709:refnum<vi>)  [unwired: 2 in, 2 out]
        n328 = property class="Pnl"(reference=w709) -> ("Controls[]"=w708:refnum<vi>[])  [unwired: 1 in, 2 out]
        n329 = property class="Pnl"(reference=w709) -> ("Decos[]"=w710:refnum<vi>[])  [unwired: 1 in, 2 out]
        n330 = for {
          tunnel: w710 -> [w714] mode=indexing
          tunnel: FALSE -> [w713]
          n331 = property class="Decor"(reference=w714, "Visible"=w713) -> ()  [unwired: 1 in, 2 out]
        }
        n332 = for {
          tunnel: w708 -> [w717] mode=indexing
          tunnel: T14."Disabled and Grayed Out" ("Disabled") -> [w716]
          tunnel: [w715] -> _
          n333 = property class="Ctl"(reference=w717, "DisabledEnum"=w716) -> (error out=w715:errorcluster)  [unwired: 1 in, 1 out]
        }
      }
      frame "Error" {
        w718 = T13[] [enum."Exit"] items=["Idle", "Init", "SetInpChan", "SetSyncDivider", "SetSyncTrg", "SetSyncOffset", "SetSyncDeadTime", "SetBinning", "SetHistoOffset", "SetHistoLen", "SetStopOvl", "SetBitShift", "SetHistoAcqTime", "GetRates", "GetAllRates", "StartMeas", "StopMeas", "AbortMeas", "GetResolution", "GetHistos", "GetAllHistos", "ReadFiFo", "WriteStatus", "Resize", "EnableControls", "DisableControls", "Error", "Exit"]
        w721 = T18 1 items=["no dialog", "OK message", "continue or stop message", "OK message + warnings", "continue/stop + warnings"] ("type of dialog (OK msg:1)")
        # "Error case: If an error occures the user is informed and the programm terminates. Add your own code to handle error events (e.g. exception lists, etc.)"
        n334 = call <vilib>:"Simple Error Handler.vi"("type of dialog (OK msg:1)"=w721, "error in (no error)"=w720) -> ()  [unwired: 3 in, 5 out]
      }
      frame "Exit" {
        n335 = Release Queue(queue=w723) -> ()  [unwired: 2 in, 3 out]
        n336 = Release Queue(queue=w722) -> ()  [unwired: 2 in, 3 out]
        n337 = Unbundle By Name(w727) -> ("DevIdx"=w726:i32)
        n338 = call "MH_CloseDevice.vi"("devidx"=w726) -> ("error out"=w725:errorcluster)  [unwired: 9 in, 1 out]
      }
    }
    n339 = call "MH_EnQError.vi"("error in (no error)"=w24, "Cmds_in"=w22) -> ("error out"=w23:errorcluster, "Cmds_out"=w21:T13[])  [unwired: 8 in]
  }
  n340 = call "MH_DataProcThread.vi"("MH_VisThread_QRef"=w7, "MH_DataProcThread_QRef"=w1) -> ()  [unwired: 10 in]
  n341 = while {
    tunnel: w7 -> [w736]
    shift-right: [w732] -> _
    shift-left: T5 {"Resol"=0.0, "DeltaT"=0.0, "NumChannels"=0} -> [w733]
    tunnel: w1 -> [w731]
    stop <- w729 stop-if-true
    # "VisualizationThread"
    n342 = Dequeue Element(queue=w736, timeout in ms (-1)=100) -> (element=w734:T6, error out=w729:errorcluster)  [unwired: 1 in, 2 out]
    n343 = Unbundle By Name(w734) -> ("Cmd"=w735:T7)
    n344 = case shown="\"TTrace\"" w735 {
      tunnel: w734 -> [_ w749 w751 w763 w771 w775 w779]
      tunnel: w733 -> [w739 w747 w753 w755 w770 w774 w778]
      tunnel: [w739 w747 w752 w755 w770 w773 w777] -> w732
      tunnel: w731 -> [w738 _ _ _ w767 _ _]
      tunnel: w729 -> [w737 _ _ _ _ _ _]
      frame "_none_", Default {
        n345 = case shown="No Error" w737 {
          tunnel: w738 -> [w743 _]
          frame No Error {
            n346 = Get Queue Status(queue=w743) -> (# elements in queue=w741:i32)  [unwired: 2 in, 7 out]
            n347 = Format Into String(format string="Elements in Q: %d", w741) -> (resulting string=w740:string)  [unwired: 2 in, 1 out]
            n348 = local write "Status"(w740) -> ()
          }
          frame Error {
          }
        }
      }
      frame "Histo" {
        n349 = Unbundle By Name(w749) -> ("Histos"=w744:u32[][])
        n350 = Unbundle By Name(w747) -> ("Resol"=w746:dbl)
        n351 = Bundle(0.0, "Resol"=w746, "Histos"=w744) -> (→"HistoGraph":cluster{dbl, "Resol":dbl, "Histos":u32[][]})  [unwired: 1 in]
      }
      frame "nChannels" {
        n352 = Unbundle By Name(w751) -> ("nChannels"=w750:i32)
        n353 = Bundle By Name(cluster=w753, "NumChannels"=w750) -> (w752:T5)
      }
      frame "TTrace" {
        n354 = Unbundle By Name(w763) -> ("Total bin"=w762:u64, "Bin"=w761:i32, "TimeTrace"=w760:u32[][])
        n355 = Unbundle By Name(w755) -> ("DeltaT"=w754:dbl)
        n356 = call "MH_TTraceToGraph.vi"("DeltaT"=w754, "TimeTrace"=w760, "Bin"=w761, "Total bin"=w762) -> ("TimeTrace_out"=w757:u32[][], "dt"=w758:dbl, "T0"=w759:dbl)  [unwired: 5 in]
        n357 = Bundle("T0"=w759, "dt"=w758, "TimeTrace_out"=w757) -> (→"TTraceGraph":T19)  [unwired: 1 in]
      }
      frame "Status" {
        n358 = Unbundle By Name(w771) -> ("Status"=w768:string)
        n359 = Get Queue Status(queue=w767) -> (# elements in queue=w766:i32)  [unwired: 2 in, 7 out]
        n360 = Format Into String(format string="\t\tElements in Q: %d", w766) -> (resulting string=w764:string)  [unwired: 2 in, 1 out]
        n361 = Concatenate Strings(w768, w764) -> (w769:string)
        n362 = local write "Status"(w769) -> ()
      }
      frame "DeltaT" {
        n363 = Unbundle By Name(w775) -> ("DeltaT"=w772:dbl)
        n364 = Bundle By Name(cluster=w774, "DeltaT"=w772) -> (w773:T5)
      }
      frame "Resol" {
        n365 = Unbundle By Name(w779) -> ("Resol"=w776:dbl)
        n366 = Bundle By Name(cluster=w778, "Resol"=w776) -> (w777:T5)
      }
    }
  }
